vi "Autonomous Independent.vi"() -> ()   [LabVIEW 2020]
doc: "This VI is called when autonomous begins, and will automatically be terminated when autonomous ends. You can carry out timed or sensor driven robot movement independently without needing to return to the caller."
uses:
  <vilib>/Rock Robotics/WPI/ThirdParty/Phoenix-LabVIEW/Motor Controller/Controls/CTRE_Phoenix_MotorControl_ControlMode.ctl
  <vilib>/Rock Robotics/WPI/SafetyOutput/WPI_SafetyOutputConfigMenu.ctl
  <vilib>/Rock Robotics/WPI/Solenoid/WPI_SolenoidValue.ctl
  <vilib>/Rock Robotics/WPI/Utilities/WPI_GetSetVariantRefNum.vi
  <vilib>/Rock Robotics/Network Tables/NT Read String.vi
  <vilib>/Rock Robotics/Network Tables/NT Write Numeric Array.vi
  <vilib>/Rock Robotics/WPI/RobotDrive/WPI_RobotDriveMecanumDrive_Cartesian.vi
  <vilib>/Rock Robotics/WPI/Solenoid/WPI_SolenoidSetEnum.vi
panel:
  out "Current Movement, for debugging":T1={"X Joystick Value"=0.0, "Y Joystick Value"=-0.25, "Delay (sec)"=2.0, "Movement Name"="Drive Forwad", "Z Joystick Value "=0.0} {"Y Joystick Value" scale=1.0..-1.0; "X Joystick Value" scale=-1.0..1.0}
  in  "Array of robot movements":T2(array[cluster])=[{"X Joystick Value"=0.0, "Y Joystick Value"=0.25, "Delay (sec)"=1.0, "Movement Name"="Go Back", "Z Joystick Value"=0.0}, {"X Joystick Value"=0.0, "Y Joystick Value"=0.0, "Delay (sec)"=3.0, "Movement Name"="STOP", "Z Joystick Value"=0.0}, {"X Joystick Value"=0.0, "Y Joystick Value"=-0.25, "Delay (sec)"=2.0, "Movement Name"="Drive Forwad", "Z Joystick Value"=0.0}]
  # "Be sure to right-click and choose Data Operations>>Make Current Value default if you want to save the array values with the VI"
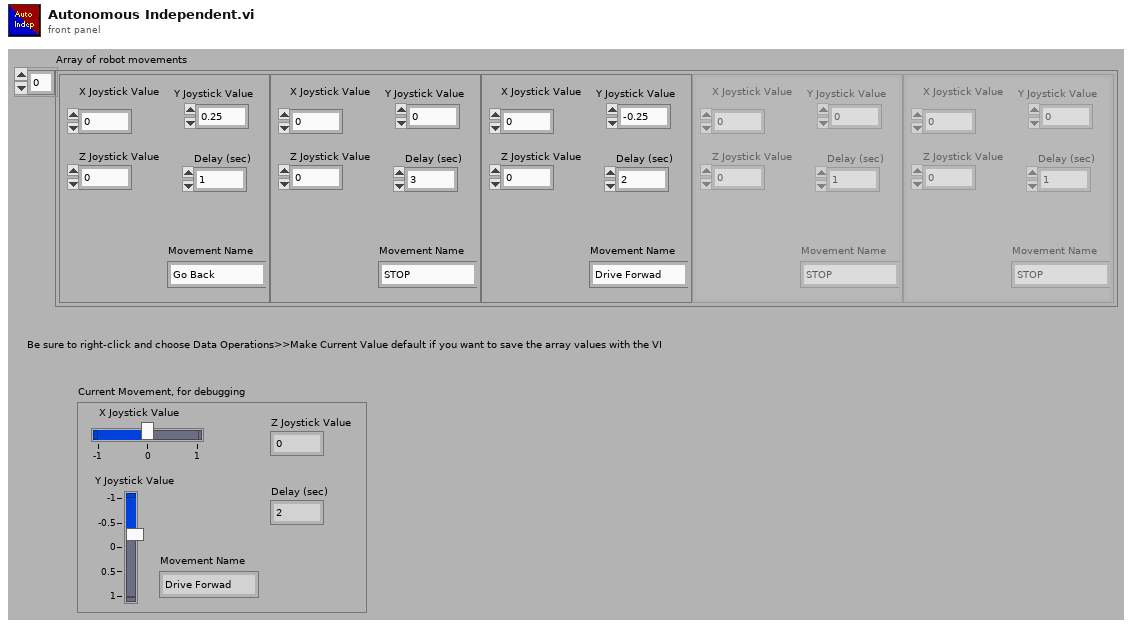
[diagram p1: front panel]
types:
  T1 = cluster{"X Joystick Value":dbl, "Y Joystick Value":dbl, "Delay (sec)":dbl, "Movement Name":string, "Z Joystick Value ":dbl}
  T2 = cluster{"X Joystick Value":dbl, "Y Joystick Value":dbl, "Delay (sec)":dbl, "Movement Name":string, "Z Joystick Value":dbl}[]
  T3 = typedef "WPI_JoystickDevRef.ctl" = cluster{"Device":T4}
  T4 = typedef "WPI_JoystickDeviceEnum.ctl" = enum16{"USB 0", "USB 1", "USB 2", "USB 3", "USB 4", "USB 5"}
  T5 = typedef "WPI_SafetyOutputConfigMenu.ctl" = enum16{"Enable", "Disable"}
  T6 = typedef "WPI_SolenoidValue.ctl" = enum16{"Off", "On", "Forward", "Reverse"}
  T7 = typedef "WPI_MotorControlDeviceRef.ctl" = cluster{"DeviceStatus":errorcluster, "Type":T8, "PWM":cluster{"PWM Channel":T9, "DeadBand":T10}, "CAN":cluster{"Device Number":u8, "SetOutput VI Ref":variant, "GetOutput VI Ref":variant, "Enable VI Ref":variant, "Disable VI Ref":variant, "Data":variant}, "Invert":bool, "DIO PWM":cluster{"PWM \"Enable\" Channel":T9, "DIOChannel":T11, "PWM Rate":dbl}}
  T8 = typedef "WPI_MotorControlType.ctl" = enum16{"PWM", "CAN", "DIO PWM"}
  T9 = typedef "FPGA_DIOPWMChannel.ctl" = enum8{"PWM 0", "PWM 1", "PWM 2", "PWM 3", "PWM 4", "PWM 5", "PWM 6", "PWM 7", "PWM 8", "PWM 9", "PWM MXP 0", "PWM MXP 1", "PWM MXP 2", "PWM MXP 3", "PWM MXP 4", "PWM MXP 5", "PWM MXP 6", "PWM MXP 7", "PWM MXP 8", "PWM MXP 9", "Invalid"}
  T10 = typedef "WPI_PWMDeadband.ctl" = cluster{"Name":string, "maxPositivePwm":i32, "minPositivePwm":i32, "centerPwm":i32, "maxNegativePwm":i32, "minNegativePwm":i32, "angularRange":u16}
  T11 = typedef "FPGA_DIOChannel.ctl" = enum8{"DIO 0", "DIO 1", "DIO 2", "DIO 3", "DIO 4", "DIO 5", "DIO 6", "DIO 7", "DIO 8", "DIO 9", "DIO MXP 0", "DIO MXP 1", "DIO MXP 2", "DIO MXP 3", "DIO MXP 4", "DIO MXP 5", "DIO MXP 6", "DIO MXP 7", "DIO MXP 8", "DIO MXP 9", "DIO MXP 10", "DIO MXP 11", "DIO MXP 12", "DIO MXP 13", "DIO MXP 14", "DIO MXP 15", "SPI Port CS1", "SPI Port CS2", "SPI Port CS3", "SPI Port MISO", "SPI Port MOSI", "Invalid"}
  T12 = typedef "WPI_RobotDriveDevRef.ctl" = cluster{"DevStatus":errorcluster, "Motors[]":T7[], "Square Inputs":bool, "Max Output":dbl}
  T13 = typedef "CTRE_Phoenix_MotorControl_ControlMode.ctl" = u16
  T14 = typedef "WPI_EncoderDevRef.ctl" = cluster{"DevStatus":errorcluster, "EncoderIndex":T15, "CounterIndex":T16, "DistancePerCount":dbl, "Decoding Type":T17}
  T15 = typedef "FPGA_EncoderIdx.ctl" = enum8{"Enc 0", "Enc 1", "Enc 2", "Enc 3", "Enc 4", "Enc 5", "Enc 6", "Enc 7", "Invalid"}
  T16 = typedef "FPGA_CounterCtrSystemIndex.ctl" = enum8{"Ctr 0", "Ctr 1", "Ctr 2", "Ctr 3", "Ctr 4", "Ctr 5", "Ctr 6", "Ctr 7", "Invalid"}
  T17 = typedef "WPI_EncoderType.ctl" = enum16{"1x", "2x", "4x"}
  T18 = typedef "WPI_SolenoidDevRef.ctl" = cluster{"DevStatus":errorcluster, "Pneumatics Control Module":u8, "Forward Solenoid Channel":T19, "Reverse Solenoid Channel":T19}
  T19 = typedef "WPI_SolenoidChannel.ctl" = enum8{"Solenoid 0", "Solenoid 1", "Solenoid 2", "Solenoid 3", "Solenoid 4", "Solenoid 5", "Solenoid 6", "Solenoid 7", "Solenoid 8", "Solenoid 9", "Solenoid 10", "Solenoid 11", "Solenoid 12", "Solenoid 13", "Solenoid 14", "Solenoid 15", "Invalid"}
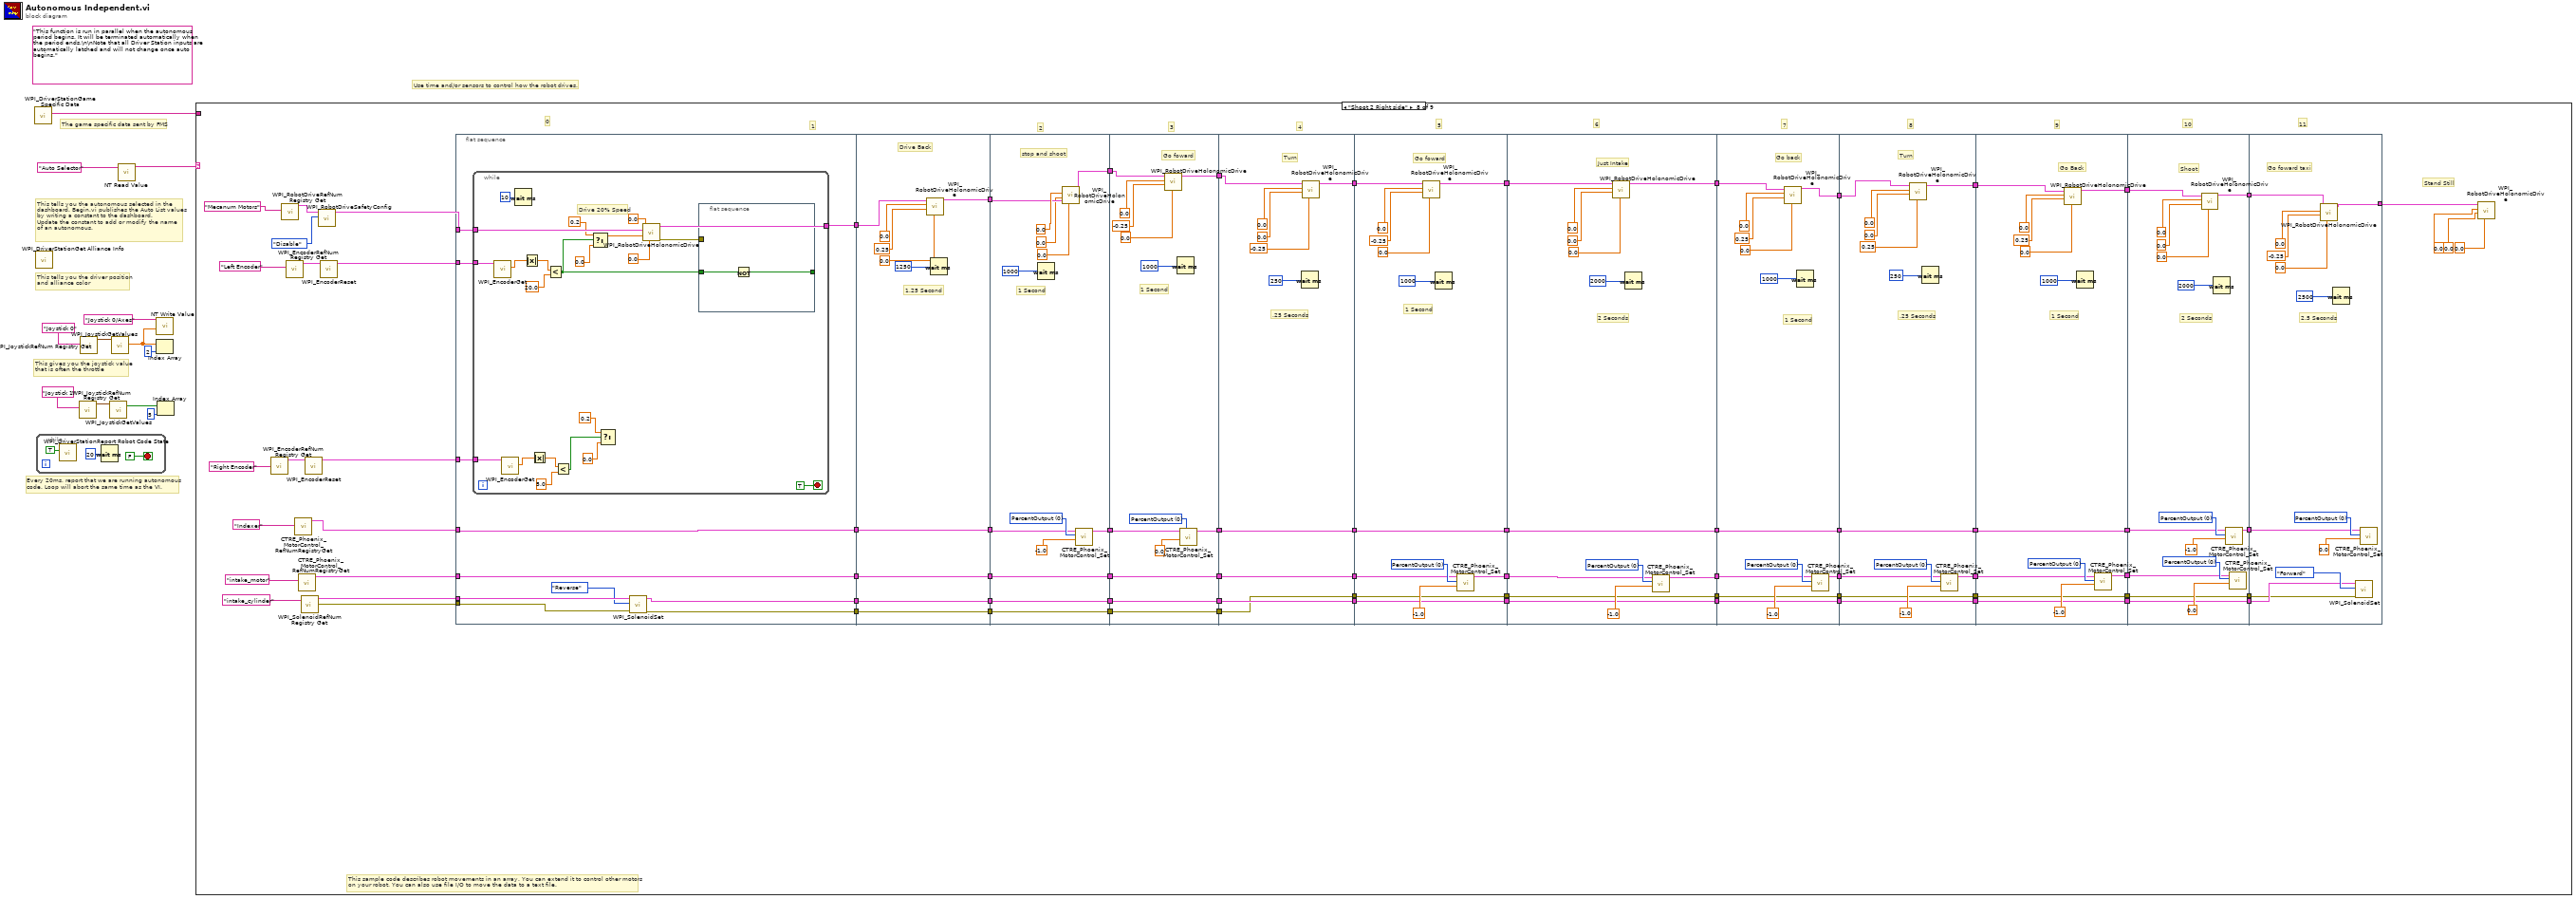
[diagram p0: block diagram]
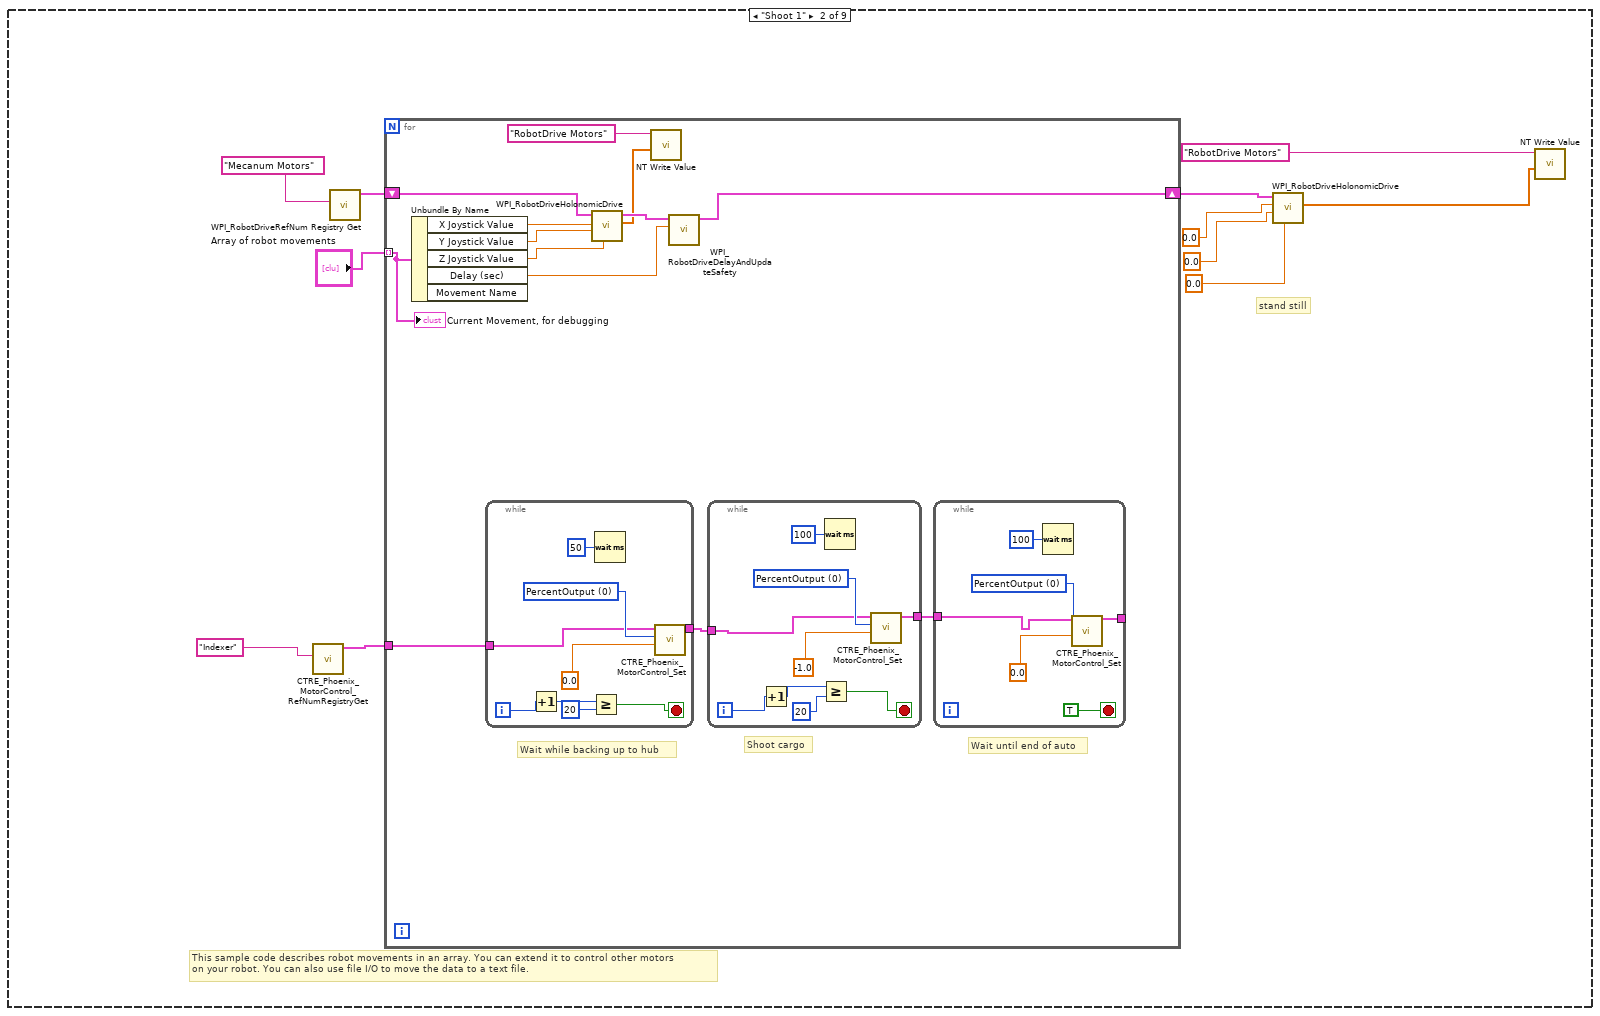
[diagram p3: hidden frame]
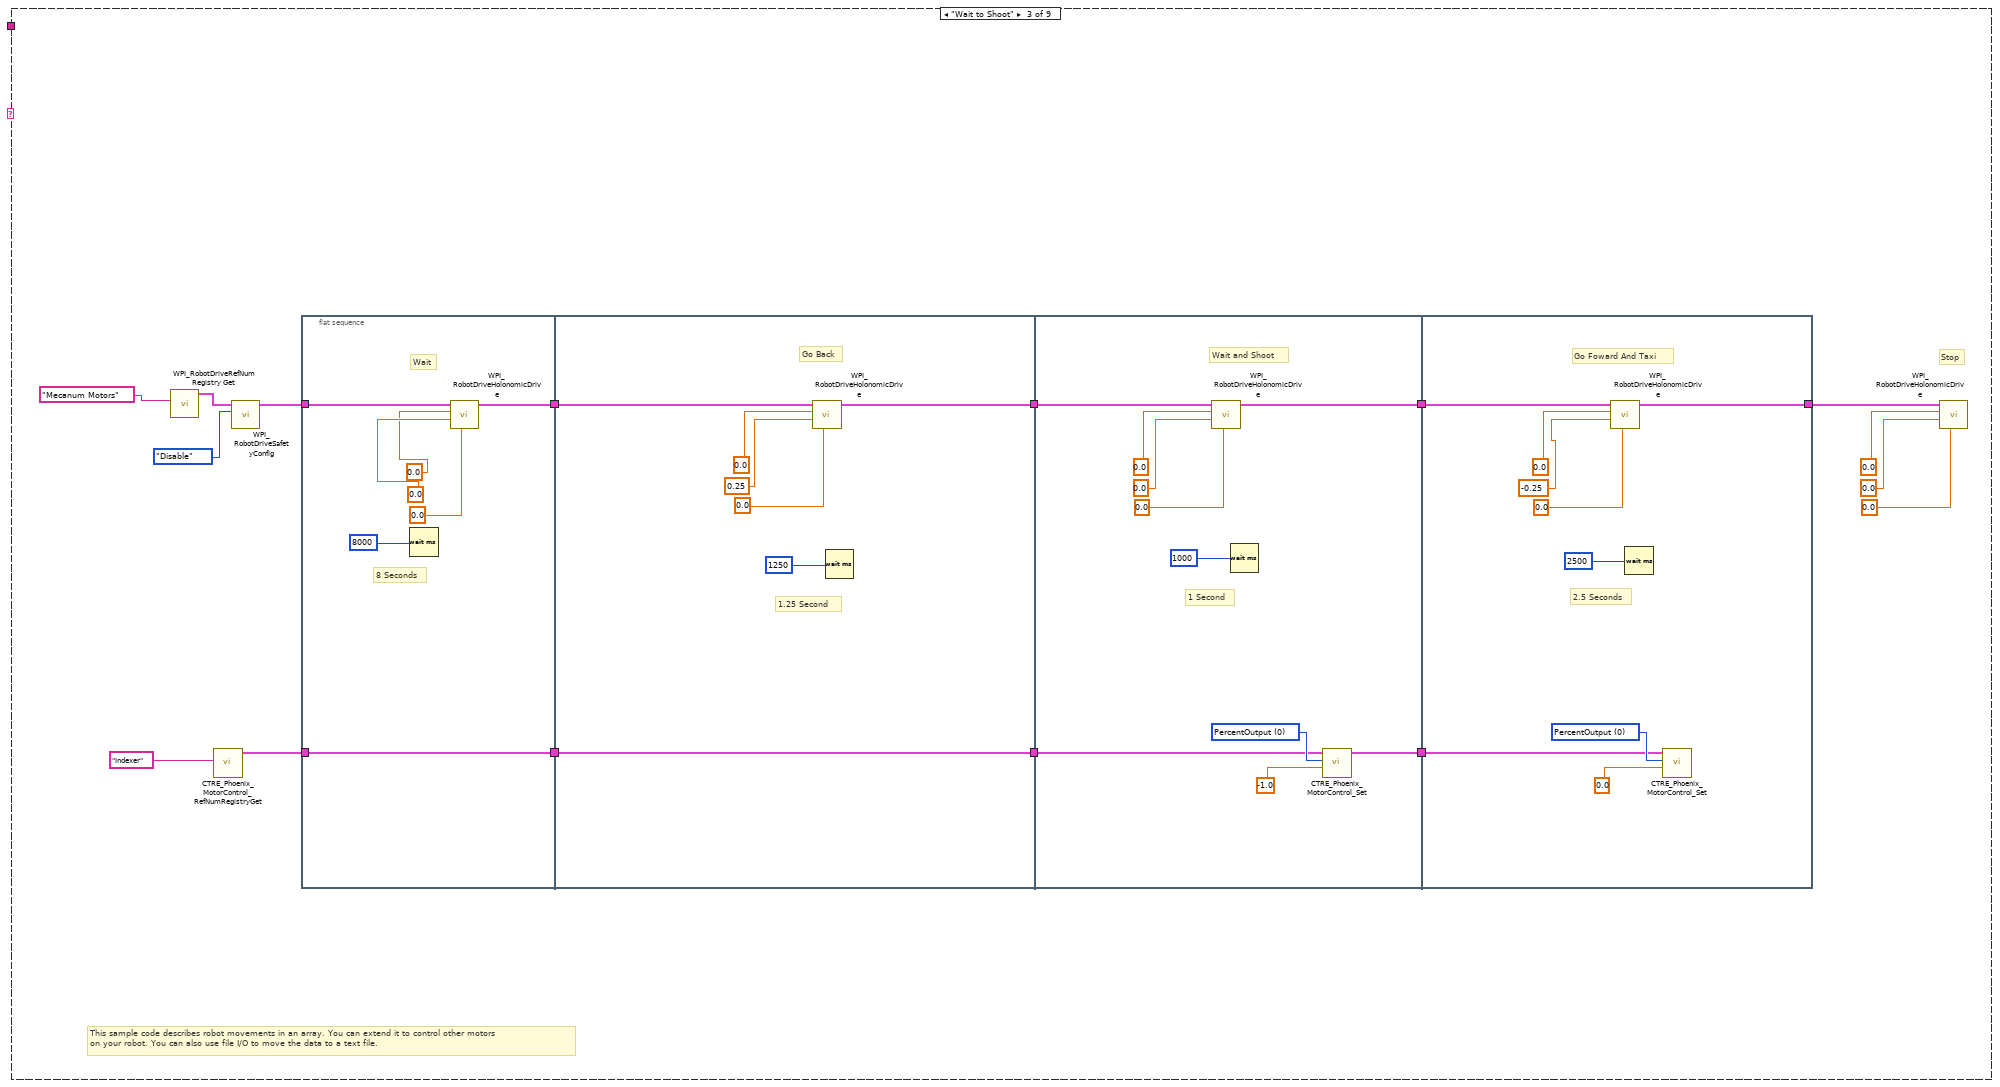
[diagram p4: hidden frame]
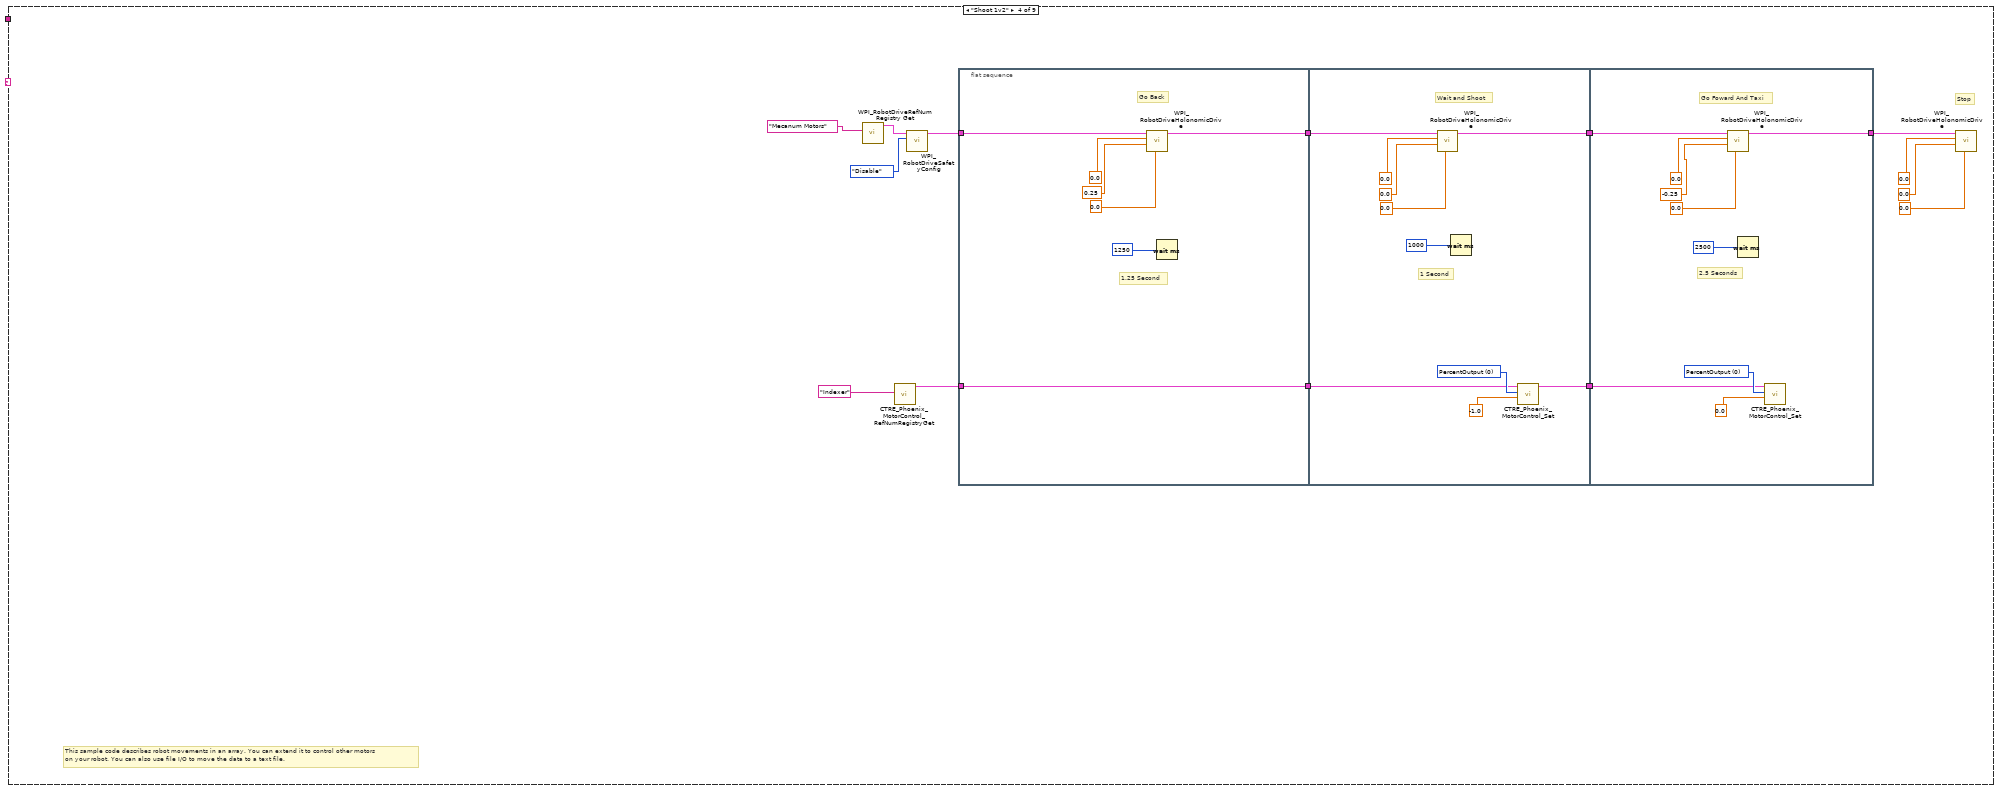
[diagram p5: hidden frame]
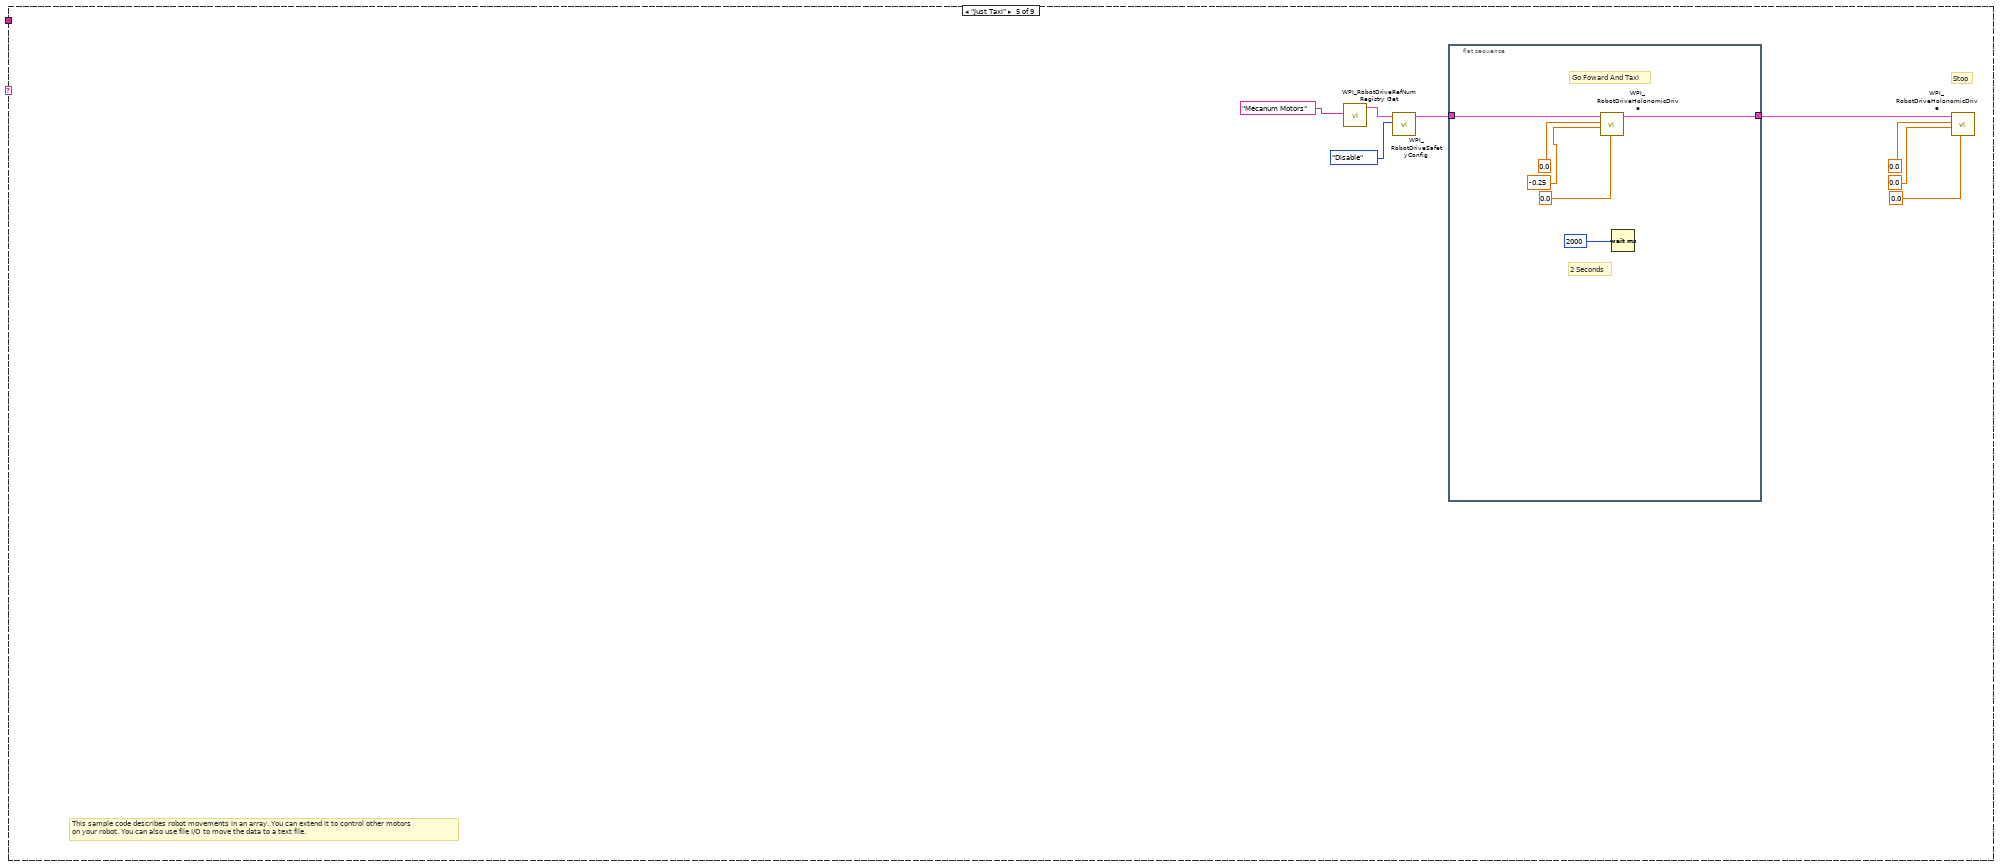
[diagram p6: hidden frame]
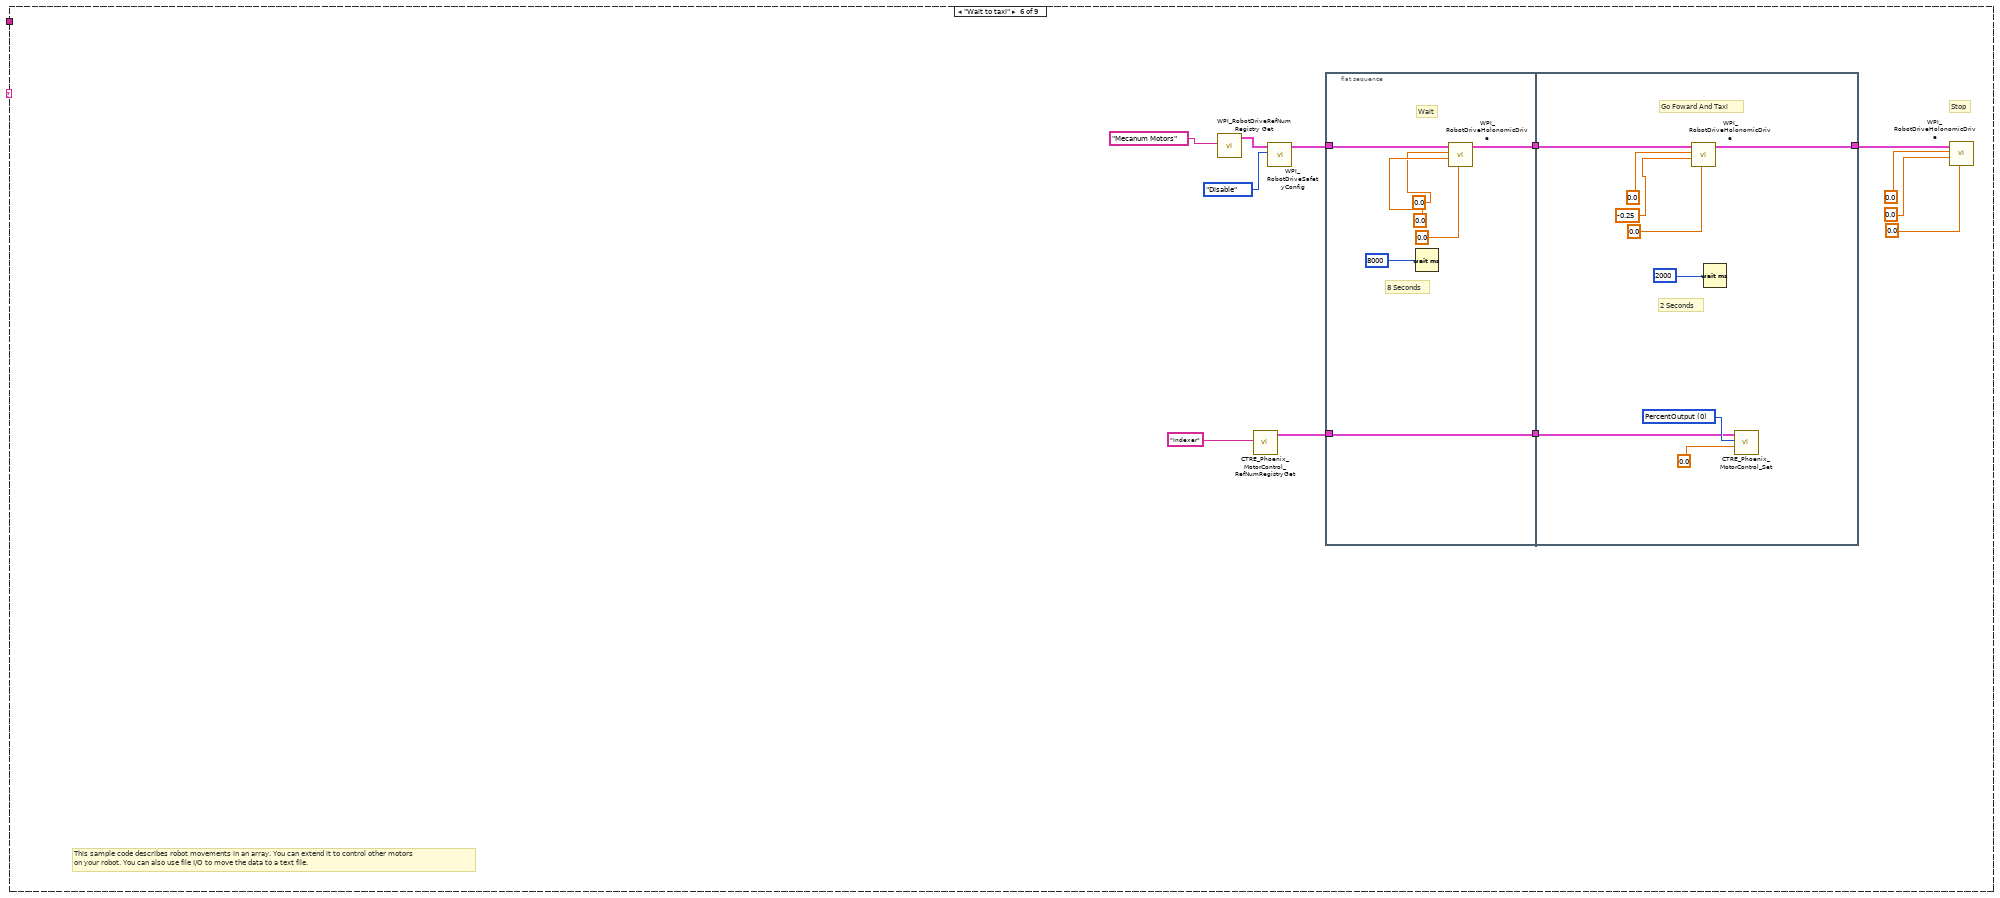
[diagram p7: hidden frame]
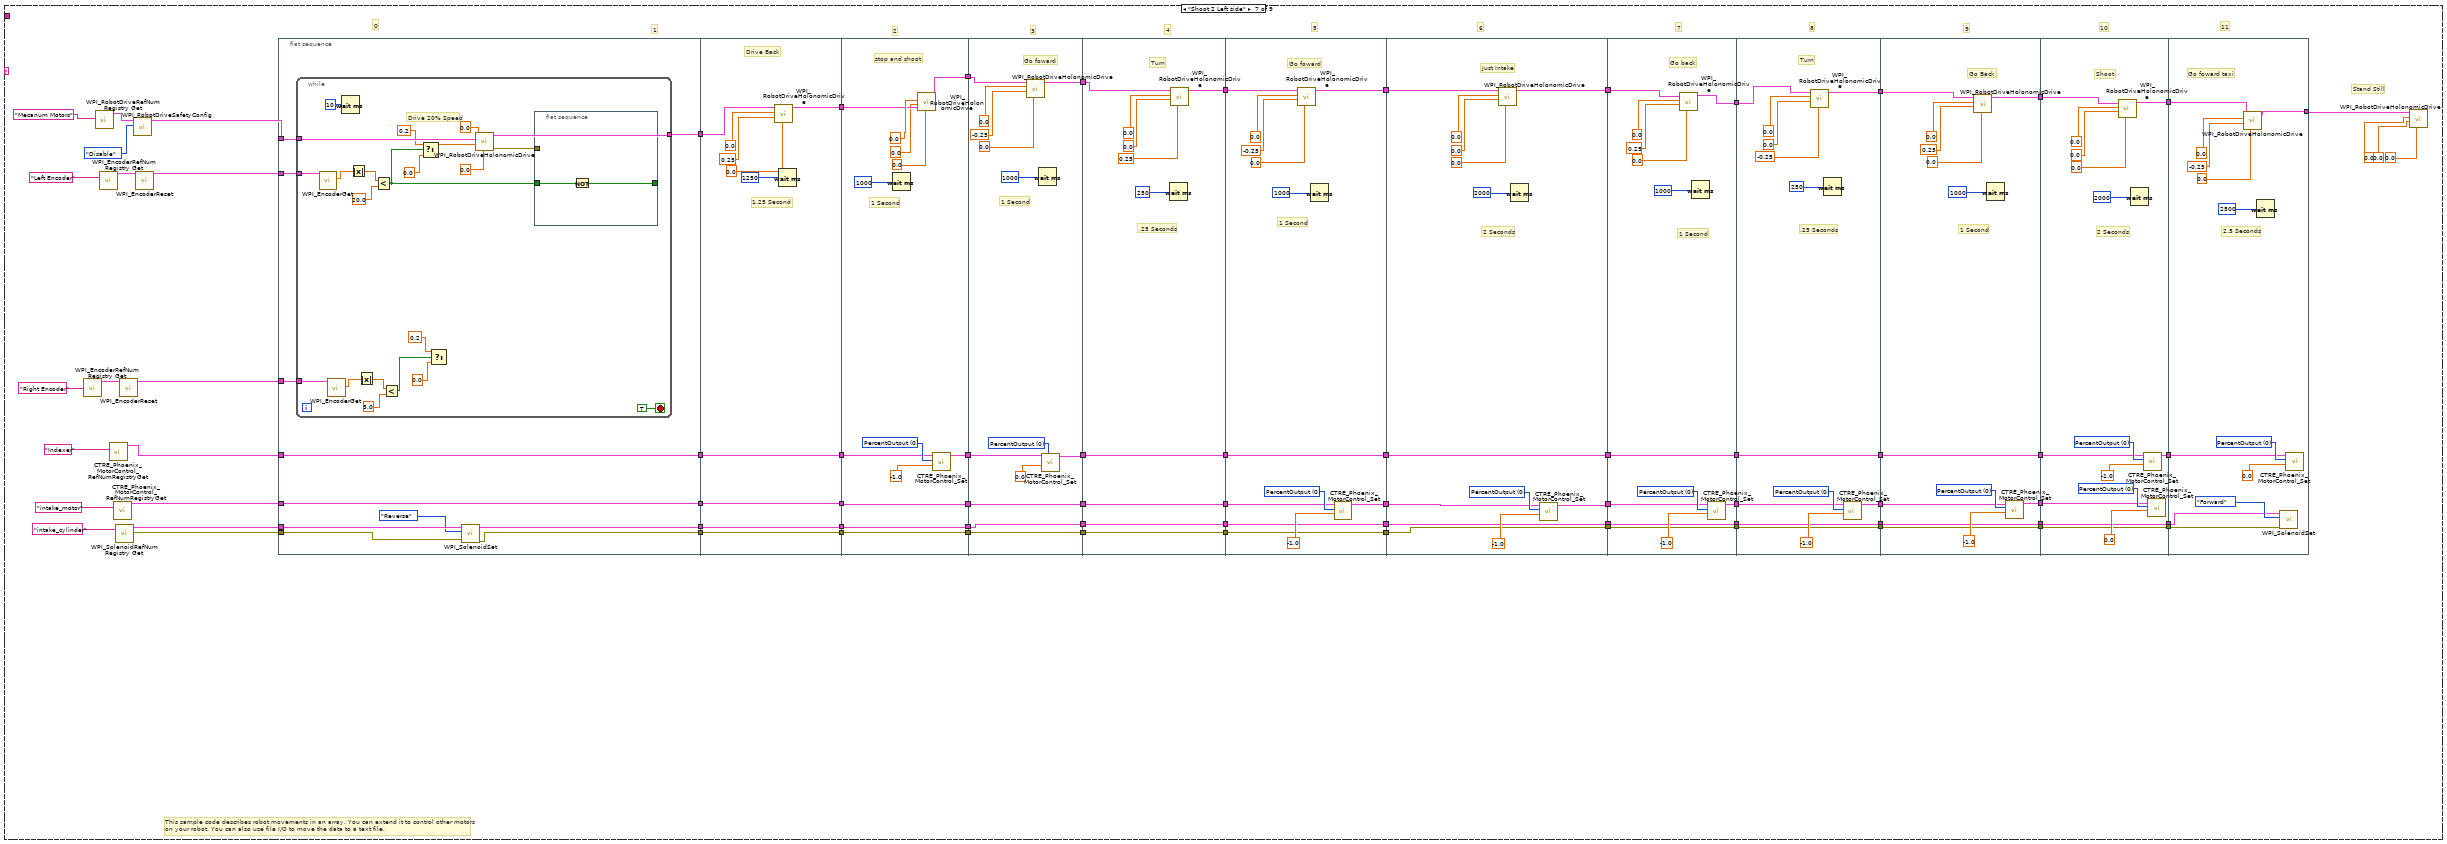
[diagram p8: hidden frame]
diagram:
  (unwired) "This function is run in parallel when the autonomous period begins. It will be terminated automatically when the period ends.\n\nNote that all Driver Station inputs are automatically latched and will not change once auto begins."
  # "The game specific data sent by FMS"
  # "This tells you the autonomous selected in the \ndashboard. Begin.vi publishes the Auto List values\nby writing a constant to the dashboard.\nUpdate the constant to add or modify the name\nof an autonomous."
  # "Every 20ms, report that we are running autonomous\ncode. Loop will abort the same time as the VI."
  # "This gives you the joystick value\nthat is often the throttle"
  # "Use time and/or sensors to control how the robot drives."
  # "This tells you the driver position\nand alliance color"
  n1 = call <vilib>:"WPI_DriverStationGame Specific Data.vi"() -> ("Game Specific Data"=w6:string)  [unwired: 11 in]
  n2 = call <vilib>:"WPI_DriverStationGet Alliance Info.vi"() -> ()  [unwired: 12 out]
  n3 = while {
    stop <- FALSE stop-if-true
    n4 = call <vilib>:"WPI_DriverStationReport Robot Code State.vi"("Autonomous"=TRUE) -> ()  [unwired: 10 in, 1 out]
    n5 = Wait (ms)(milliseconds to wait=u32 20) -> ()  [unwired: 1 out]
  }
  n6 = call <vilib>:"WPI_JoystickRefNum Registry Get.vi"("refnum name"="Joystick 1") -> ("JoystickDevRef"=w5:T3)  [unwired: 1 in, 9 out]
  n7 = call <vilib>:"WPI_JoystickRefNum Registry Get.vi"("refnum name"="Joystick 0") -> ("JoystickDevRef"=w11:T3)  [unwired: 1 in, 9 out]
  n8 = call <vilib>:"WPI_JoystickGetValues.vi"("JoystickDevRef"=w5) -> ("Buttons"=w1:bool[])  [unwired: 6 in, 4 out]
  n9 = call <vilib>:"WPI_JoystickGetValues.vi"("JoystickDevRef"=w11) -> ("Axes"=w8:dbl[])  [unwired: 6 in, 4 out]
  n10 = call-poly <vilib>:"NT Read Value.vi"("Name"="Auto Selector") -> ("String"=w2:string)  [unwired: 9 in, 1 out]
  n11 = call-poly <vilib>:"NT Write Value.vi"("Numeric Array"=w8, "Name"="Joystick 0/Axes") -> ()  [unwired: 9 in, 1 out]
  n12 = Index Array(array=w8, index=2) -> ()  [unwired: 1 out]
  n13 = Index Array(array=w1, index=5) -> ()  [unwired: 1 out]
  n14 = case shown="\"Shoot 2 Right side\"" w2 {
    tunnel: w6 -> [_ _ _ _ _ _ _ _ _]
    frame Default {
      # "You can put your main auto here, or you can right-click on the case and make any\nother frame be the default case."
      # "This is the frame that will execute if no selection is made, or if it is not recognized"
    }
    frame "Shoot 1" {
      # "stand still"
      # "This sample code describes robot movements in an array. You can extend it to control other motors\non your robot. You can also use file I/O to move the data to a text file."
      n15 = call <vilib>:"CTRE_Phoenix_MotorControl_RefNumRegistryGet.vi"("refnum name"="Indexer") -> ("PhoenixMotorControlDevRef"=w16:T7)  [unwired: 9 in, 1 out]
      n16 = call <vilib>:"WPI_RobotDriveRefNum Registry Get.vi"("refnum name"="Mecanum Motors") -> ("RobotDriveDevRef"=w26:T12)  [unwired: 1 in, 9 out]
      n17 = for {
        shift-right: [w38] -> w22
        shift-left: w26 -> [w30]
        tunnel: "Array of robot movements" -> [w34] mode=indexing
        tunnel: w16 -> [w29]
        # "Wait until end of auto"
        # "Shoot cargo"
        # "Wait while backing up to hub"
        n18 = Unbundle By Name "Unbundle By Name"(w34) -> ("X Joystick Value"=w37:dbl, "Y Joystick Value"=w36:dbl, "Z Joystick Value"=w31:dbl, "Delay (sec)"=w35:dbl)  [unwired: 1 out]
        n19 = while {
          tunnel: w29 -> [w62]
          tunnel: [w55] -> w28
          i -> [w60]
          stop <- w58 stop-if-true
          w63 = T13 0 items=["PercentOutput"=0, "Position"=1, "Velocity"=2, "Current"=3, "Follower"=5, "MotionProfile"=6, "MotionMagic"=7, "MotionProfileArc"=10, "Disabled"=15] ("Control Mode")
          n20 = Increment(x=w60) -> (x+1=w59:i32)
          n21 = Greater Or Equal?(x=w59, y=20) -> (x >= y?=w58:bool)
          n22 = Wait (ms)(milliseconds to wait=u32 50) -> ()  [unwired: 1 out]
          n23 = call <vilib>:"CTRE_Phoenix_MotorControl_Set.vi"("Output"=0.0, "Control Mode"=w63, "PhoenixMotorControlDevRef"=w62) -> ("PhoenixMotorControlDevRef"=w55:T7)  [unwired: 7 in, 1 out]
        }
        n24 = call-poly <vilib>:"WPI_RobotDriveHolonomicDrive.vi"("Rotation"=w31, "Y"=w36, "X"=w37, "RobotDriveDevRef"=w30) -> ("Motor Values"=w32:dbl[], "RobotDriveDevRef"=w39:T12)  [unwired: 5 in, 1 out]
        n25 = call-poly <vilib>:"NT Write Value.vi"("Numeric Array"=w32, "Name"="RobotDrive Motors") -> ()  [unwired: 9 in, 1 out]
        n26 = call <vilib>:"WPI_RobotDriveDelayAndUpdateSafety.vi"("Delay (s)"=w35, "RobotDriveDevRef"=w39) -> ("RobotDriveDevRef 2"=w38:T12)  [unwired: 8 in, 1 out]
        n27 = while {
          tunnel: w28 -> [w50]
          tunnel: [w47] -> w27
          i -> [w49]
          stop <- w48 stop-if-true
          w54 = T13 0 items=["PercentOutput"=0, "Position"=1, "Velocity"=2, "Current"=3, "Follower"=5, "MotionProfile"=6, "MotionMagic"=7, "MotionProfileArc"=10, "Disabled"=15] ("Control Mode")
          n28 = Increment(x=w49) -> (x+1=w46:i32)
          n29 = Greater Or Equal?(x=w46, y=20) -> (x >= y?=w48:bool)
          n30 = Wait (ms)(milliseconds to wait=u32 100) -> ()  [unwired: 1 out]
          n31 = call <vilib>:"CTRE_Phoenix_MotorControl_Set.vi"("Output"=-1.0, "Control Mode"=w54, "PhoenixMotorControlDevRef"=w50) -> ("PhoenixMotorControlDevRef"=w47:T7)  [unwired: 7 in, 1 out]
        }
        n32 = while {
          tunnel: w27 -> [w42]
          tunnel: [w41] -> _
          stop <- TRUE stop-if-true
          w45 = T13 0 items=["PercentOutput"=0, "Position"=1, "Velocity"=2, "Current"=3, "Follower"=5, "MotionProfile"=6, "MotionMagic"=7, "MotionProfileArc"=10, "Disabled"=15] ("Control Mode")
          n33 = Wait (ms)(milliseconds to wait=u32 100) -> ()  [unwired: 1 out]
          n34 = call <vilib>:"CTRE_Phoenix_MotorControl_Set.vi"("Output"=0.0, "Control Mode"=w45, "PhoenixMotorControlDevRef"=w42) -> ("PhoenixMotorControlDevRef"=w41:T7)  [unwired: 7 in, 1 out]
        }
        "Current Movement, for debugging" <- w34
      }
      n35 = call-poly <vilib>:"WPI_RobotDriveHolonomicDrive.vi"("Rotation"=0.0 ("X axis value"), "Y"=0.0 ("X axis value"), "X"=0.0 ("X axis value"), "RobotDriveDevRef"=w22) -> ("Motor Values"=w19:dbl[])  [unwired: 5 in, 2 out]
      n36 = call-poly <vilib>:"NT Write Value.vi"("Numeric Array"=w19, "Name"="RobotDrive Motors") -> ()  [unwired: 9 in, 1 out]
    }
    frame "Wait to Shoot" {
      # "Stop"
      # "This sample code describes robot movements in an array. You can extend it to control other motors\non your robot. You can also use file I/O to move the data to a text file."
      n37 = call <vilib>:"WPI_RobotDriveRefNum Registry Get.vi"("refnum name"="Mecanum Motors") -> ("RobotDriveDevRef"=w77:T12)  [unwired: 1 in, 9 out]
      n38 = call <vilib>:"CTRE_Phoenix_MotorControl_RefNumRegistryGet.vi"("refnum name"="Indexer") -> ("PhoenixMotorControlDevRef"=w64:T7)  [unwired: 9 in, 1 out]
      n39 = call <vilib>:"WPI_RobotDriveSafetyConfig.vi"("mode"=WPI_SafetyOutputConfigMenu."Disable", "RobotDriveDevRef"=w77) -> ("RobotDriveDevRef"=w76:T12)  [unwired: 8 in, 1 out]
      n40 = flat-sequence {
        tunnel: w76 -> [w82]
        tunnel: [w81] -> w75
        tunnel: [w80] -> w65
        tunnel: w64 -> [w80]
        tunnel: w75 -> [w89]
        tunnel: [w88] -> w74
        tunnel: [w87] -> w66
        tunnel: w65 -> [w87]
        tunnel: w74 -> [w99]
        tunnel: [w98] -> w73
        tunnel: [w95] -> w67
        tunnel: w66 -> [w94]
        tunnel: w73 -> [w110]
        tunnel: [w109] -> w69
        tunnel: w67 -> [w106]
        frame #0 {
          # "Wait"
          # "8 Seconds"
          n41 = Wait (ms)(milliseconds to wait=u32 8000) -> ()  [unwired: 1 out]
          n42 = call-poly <vilib>:"WPI_RobotDriveHolonomicDrive.vi"("Rotation"=0.0 ("X axis value"), "Y"=0.0 ("X axis value"), "X"=0.0 ("X axis value"), "RobotDriveDevRef"=w82) -> ("RobotDriveDevRef"=w81:T12)  [unwired: 5 in, 2 out]
        }
        frame #1 {
          # "Go Back"
          # "1.25 Second"
          n43 = call-poly <vilib>:"WPI_RobotDriveHolonomicDrive.vi"("Rotation"=0.0, "Y"=0.25, "X"=0.0, "RobotDriveDevRef"=w89) -> ("RobotDriveDevRef"=w88:T12)  [unwired: 5 in, 2 out]
          n44 = Wait (ms)(milliseconds to wait=u32 1250) -> ()  [unwired: 1 out]
        }
        frame #2 {
          w97 = T13 0 items=["PercentOutput"=0, "Position"=1, "Velocity"=2, "Current"=3, "Follower"=5, "MotionProfile"=6, "MotionMagic"=7, "MotionProfileArc"=10, "Disabled"=15] ("Control Mode")
          # "Wait and Shoot"
          # "1 Second"
          n45 = call-poly <vilib>:"WPI_RobotDriveHolonomicDrive.vi"("Rotation"=0.0, "Y"=0.0, "X"=0.0, "RobotDriveDevRef"=w99) -> ("RobotDriveDevRef"=w98:T12)  [unwired: 5 in, 2 out]
          n46 = Wait (ms)(milliseconds to wait=u32 1000) -> ()  [unwired: 1 out]
          n47 = call <vilib>:"CTRE_Phoenix_MotorControl_Set.vi"("Output"=-1.0, "Control Mode"=w97, "PhoenixMotorControlDevRef"=w94) -> ("PhoenixMotorControlDevRef"=w95:T7)  [unwired: 7 in, 1 out]
        }
        frame #3 {
          w108 = T13 0 items=["PercentOutput"=0, "Position"=1, "Velocity"=2, "Current"=3, "Follower"=5, "MotionProfile"=6, "MotionMagic"=7, "MotionProfileArc"=10, "Disabled"=15] ("Control Mode")
          # "2.5 Seconds"
          # "Go Foward And Taxi"
          n48 = call-poly <vilib>:"WPI_RobotDriveHolonomicDrive.vi"("Rotation"=0.0, "Y"=-0.25, "X"=0.0, "RobotDriveDevRef"=w110) -> ("RobotDriveDevRef"=w109:T12)  [unwired: 5 in, 2 out]
          n49 = Wait (ms)(milliseconds to wait=u32 2500) -> ()  [unwired: 1 out]
          n50 = call <vilib>:"CTRE_Phoenix_MotorControl_Set.vi"("Output"=0.0, "Control Mode"=w108, "PhoenixMotorControlDevRef"=w106) -> ()  [unwired: 7 in, 2 out]
        }
      }
      n51 = call-poly <vilib>:"WPI_RobotDriveHolonomicDrive.vi"("Rotation"=0.0, "Y"=0.0, "X"=0.0, "RobotDriveDevRef"=w69) -> ()  [unwired: 5 in, 3 out]
    }
    frame "Shoot 1v2" {
      # "Stop"
      # "This sample code describes robot movements in an array. You can extend it to control other motors\non your robot. You can also use file I/O to move the data to a text file."
      n52 = call <vilib>:"WPI_RobotDriveRefNum Registry Get.vi"("refnum name"="Mecanum Motors") -> ("RobotDriveDevRef"=w124:T12)  [unwired: 1 in, 9 out]
      n53 = call <vilib>:"CTRE_Phoenix_MotorControl_RefNumRegistryGet.vi"("refnum name"="Indexer") -> ("PhoenixMotorControlDevRef"=w114:T7)  [unwired: 9 in, 1 out]
      n54 = call <vilib>:"WPI_RobotDriveSafetyConfig.vi"("mode"=WPI_SafetyOutputConfigMenu."Disable", "RobotDriveDevRef"=w124) -> ("RobotDriveDevRef"=w113:T12)  [unwired: 8 in, 1 out]
      n55 = flat-sequence {
        tunnel: [w129] -> w123
        tunnel: [w128] -> w115
        tunnel: w114 -> [w128]
        tunnel: w113 -> [w127]
        tunnel: w123 -> [w139]
        tunnel: [w138] -> w122
        tunnel: [w135] -> w116
        tunnel: w115 -> [w134]
        tunnel: w122 -> [w150]
        tunnel: [w149] -> w118
        tunnel: w116 -> [w146]
        frame #0 {
          # "Go Back"
          # "1.25 Second"
          n56 = call-poly <vilib>:"WPI_RobotDriveHolonomicDrive.vi"("Rotation"=0.0, "Y"=0.25, "X"=0.0, "RobotDriveDevRef"=w127) -> ("RobotDriveDevRef"=w129:T12)  [unwired: 5 in, 2 out]
          n57 = Wait (ms)(milliseconds to wait=u32 1250) -> ()  [unwired: 1 out]
        }
        frame #1 {
          w137 = T13 0 items=["PercentOutput"=0, "Position"=1, "Velocity"=2, "Current"=3, "Follower"=5, "MotionProfile"=6, "MotionMagic"=7, "MotionProfileArc"=10, "Disabled"=15] ("Control Mode")
          # "Wait and Shoot"
          # "1 Second"
          n58 = call-poly <vilib>:"WPI_RobotDriveHolonomicDrive.vi"("Rotation"=0.0, "Y"=0.0, "X"=0.0, "RobotDriveDevRef"=w139) -> ("RobotDriveDevRef"=w138:T12)  [unwired: 5 in, 2 out]
          n59 = Wait (ms)(milliseconds to wait=u32 1000) -> ()  [unwired: 1 out]
          n60 = call <vilib>:"CTRE_Phoenix_MotorControl_Set.vi"("Output"=-1.0, "Control Mode"=w137, "PhoenixMotorControlDevRef"=w134) -> ("PhoenixMotorControlDevRef"=w135:T7)  [unwired: 7 in, 1 out]
        }
        frame #2 {
          w148 = T13 0 items=["PercentOutput"=0, "Position"=1, "Velocity"=2, "Current"=3, "Follower"=5, "MotionProfile"=6, "MotionMagic"=7, "MotionProfileArc"=10, "Disabled"=15] ("Control Mode")
          # "2.5 Seconds"
          # "Go Foward And Taxi"
          n61 = call-poly <vilib>:"WPI_RobotDriveHolonomicDrive.vi"("Rotation"=0.0, "Y"=-0.25, "X"=0.0, "RobotDriveDevRef"=w150) -> ("RobotDriveDevRef"=w149:T12)  [unwired: 5 in, 2 out]
          n62 = Wait (ms)(milliseconds to wait=u32 2500) -> ()  [unwired: 1 out]
          n63 = call <vilib>:"CTRE_Phoenix_MotorControl_Set.vi"("Output"=0.0, "Control Mode"=w148, "PhoenixMotorControlDevRef"=w146) -> ()  [unwired: 7 in, 2 out]
        }
      }
      n64 = call-poly <vilib>:"WPI_RobotDriveHolonomicDrive.vi"("Rotation"=0.0, "Y"=0.0, "X"=0.0, "RobotDriveDevRef"=w118) -> ()  [unwired: 5 in, 3 out]
    }
    frame "Just Taxi" {
      # "Stop"
      # "This sample code describes robot movements in an array. You can extend it to control other motors\non your robot. You can also use file I/O to move the data to a text file."
      n65 = call <vilib>:"WPI_RobotDriveRefNum Registry Get.vi"("refnum name"="Mecanum Motors") -> ("RobotDriveDevRef"=w158:T12)  [unwired: 1 in, 9 out]
      n66 = call <vilib>:"WPI_RobotDriveSafetyConfig.vi"("mode"=WPI_SafetyOutputConfigMenu."Disable", "RobotDriveDevRef"=w158) -> ("RobotDriveDevRef"=w153:T12)  [unwired: 8 in, 1 out]
      n67 = flat-sequence {
        tunnel: [w164] -> w154
        tunnel: w153 -> [w161]
        frame #0 {
          # "2 Seconds"
          # "Go Foward And Taxi"
          n68 = call-poly <vilib>:"WPI_RobotDriveHolonomicDrive.vi"("Rotation"=0.0, "Y"=-0.25, "X"=0.0, "RobotDriveDevRef"=w161) -> ("RobotDriveDevRef"=w164:T12)  [unwired: 5 in, 2 out]
          n69 = Wait (ms)(milliseconds to wait=u32 2000) -> ()  [unwired: 1 out]
        }
      }
      n70 = call-poly <vilib>:"WPI_RobotDriveHolonomicDrive.vi"("Rotation"=0.0, "Y"=0.0, "X"=0.0, "RobotDriveDevRef"=w154) -> ()  [unwired: 5 in, 3 out]
    }
    frame "Wait to taxi" {
      # "Stop"
      # "This sample code describes robot movements in an array. You can extend it to control other motors\non your robot. You can also use file I/O to move the data to a text file."
      n71 = call <vilib>:"WPI_RobotDriveRefNum Registry Get.vi"("refnum name"="Mecanum Motors") -> ("RobotDriveDevRef"=w176:T12)  [unwired: 1 in, 9 out]
      n72 = call <vilib>:"CTRE_Phoenix_MotorControl_RefNumRegistryGet.vi"("refnum name"="Indexer") -> ("PhoenixMotorControlDevRef"=w169:T7)  [unwired: 9 in, 1 out]
      n73 = call <vilib>:"WPI_RobotDriveSafetyConfig.vi"("mode"=WPI_SafetyOutputConfigMenu."Disable", "RobotDriveDevRef"=w176) -> ("RobotDriveDevRef"=w175:T12)  [unwired: 8 in, 1 out]
      n74 = flat-sequence {
        tunnel: w175 -> [w181]
        tunnel: w169 -> [w179]
        tunnel: [w180] -> w168
        tunnel: [w179] -> w167
        tunnel: [w192] -> w171
        tunnel: w168 -> [w187]
        tunnel: w167 -> [w186]
        frame #0 {
          # "Wait"
          # "8 Seconds"
          n75 = Wait (ms)(milliseconds to wait=u32 8000) -> ()  [unwired: 1 out]
          n76 = call-poly <vilib>:"WPI_RobotDriveHolonomicDrive.vi"("Rotation"=0.0 ("X axis value"), "Y"=0.0 ("X axis value"), "X"=0.0 ("X axis value"), "RobotDriveDevRef"=w181) -> ("RobotDriveDevRef"=w180:T12)  [unwired: 5 in, 2 out]
        }
        frame #1 {
          w191 = T13 0 items=["PercentOutput"=0, "Position"=1, "Velocity"=2, "Current"=3, "Follower"=5, "MotionProfile"=6, "MotionMagic"=7, "MotionProfileArc"=10, "Disabled"=15] ("Control Mode")
          # "2 Seconds"
          # "Go Foward And Taxi"
          n77 = call-poly <vilib>:"WPI_RobotDriveHolonomicDrive.vi"("Rotation"=0.0, "Y"=-0.25, "X"=0.0, "RobotDriveDevRef"=w187) -> ("RobotDriveDevRef"=w192:T12)  [unwired: 5 in, 2 out]
          n78 = Wait (ms)(milliseconds to wait=u32 2000) -> ()  [unwired: 1 out]
          n79 = call <vilib>:"CTRE_Phoenix_MotorControl_Set.vi"("Output"=0.0, "Control Mode"=w191, "PhoenixMotorControlDevRef"=w186) -> ()  [unwired: 7 in, 2 out]
        }
      }
      n80 = call-poly <vilib>:"WPI_RobotDriveHolonomicDrive.vi"("Rotation"=0.0, "Y"=0.0, "X"=0.0, "RobotDriveDevRef"=w171) -> ()  [unwired: 5 in, 3 out]
    }
    frame "Shoot 2 Left side" {
      # "11"
      # "0"
      # "Stand Still"
      # "10"
      # "9"
      # "8"
      # "7"
      # "6"
      # "5"
      # "4"
      # "3"
      # "2"
      # "1"
      # "This sample code describes robot movements in an array. You can extend it to control other motors\non your robot. You can also use file I/O to move the data to a text file."
      n81 = call <vilib>:"WPI_EncoderRefNum Registry Get.vi"("refnum name"="Right Encoder") -> ("EncoderDevRef"=w235:T14)  [unwired: 9 in, 1 out]
      n82 = call <vilib>:"WPI_RobotDriveRefNum Registry Get.vi"("refnum name"="Mecanum Motors") -> ("RobotDriveDevRef"=w238:T12)  [unwired: 1 in, 9 out]
      n83 = call <vilib>:"WPI_EncoderRefNum Registry Get.vi"("refnum name"="Left Encoder") -> ("EncoderDevRef"=w243:T14)  [unwired: 9 in, 1 out]
      n84 = call <vilib>:"CTRE_Phoenix_MotorControl_RefNumRegistryGet.vi"("refnum name"="Indexer") -> ("PhoenixMotorControlDevRef"=w265:T7)  [unwired: 9 in, 1 out]
      n85 = call <vilib>:"CTRE_Phoenix_MotorControl_RefNumRegistryGet.vi"("refnum name"="intake_motor") -> ("PhoenixMotorControlDevRef"=w262:T7)  [unwired: 9 in, 1 out]
      n86 = call <vilib>:"WPI_SolenoidRefNum Registry Get.vi"("refnum name"="intake_cylinder") -> ("error out"=w227:errorcluster, "SolenoidDevRef"=w225:T18)  [unwired: 9 in]
      n87 = call <vilib>:"WPI_EncoderReset.vi"("EncoderDevRef"=w235) -> ("EncoderDevRef"=w234:T14)  [unwired: 9 in, 1 out]
      n88 = call <vilib>:"WPI_RobotDriveSafetyConfig.vi"("mode"=WPI_SafetyOutputConfigMenu."Disable", "RobotDriveDevRef"=w238) -> ("RobotDriveDevRef"=w237:T12)  [unwired: 8 in, 1 out]
      n89 = call <vilib>:"WPI_EncoderReset.vi"("EncoderDevRef"=w243) -> ("EncoderDevRef"=w242:T14)  [unwired: 9 in, 1 out]
      n90 = flat-sequence {
        tunnel: w262 -> [w279]
        tunnel: w265 -> [w280]
        tunnel: [w276] -> w246
        tunnel: [w280] -> w245
        tunnel: [w279] -> w244
        tunnel: w242 -> [w278]
        tunnel: w237 -> [w277]
        tunnel: w234 -> [w275]
        tunnel: w227 -> [w274]
        tunnel: w225 -> [w273]
        tunnel: [w271] -> w206
        tunnel: [w270] -> w205
        tunnel: [w310] -> w269
        tunnel: [w308] -> w266
        tunnel: [w307] -> w263
        tunnel: w246 -> [w313]
        tunnel: w245 -> [w308]
        tunnel: w244 -> [w307]
        tunnel: [w306] -> w207
        tunnel: w206 -> [w306]
        tunnel: w205 -> [w305]
        tunnel: [w305] -> w204
        tunnel: w269 -> [w324]
        tunnel: [w323] -> w268
        tunnel: w266 -> [w319]
        tunnel: w263 -> [w317]
        tunnel: [w318] -> w250
        tunnel: [w317] -> w247
        tunnel: [w316] -> w208
        tunnel: w207 -> [w316]
        tunnel: w204 -> [w315]
        tunnel: [w315] -> w203
        tunnel: w268 -> [w337]
        tunnel: [w335] -> w261
        tunnel: [w330] -> w251
        tunnel: w250 -> [w331]
        tunnel: [w334] -> w248
        tunnel: w247 -> [w334]
        tunnel: [w329] -> w209
        tunnel: w208 -> [w329]
        tunnel: w203 -> [w328]
        tunnel: [w328] -> w202
        tunnel: w261 -> [w346]
        tunnel: [w345] -> w260
        tunnel: [w344] -> w252
        tunnel: w251 -> [w344]
        tunnel: [w343] -> w249
        tunnel: w248 -> [w343]
        tunnel: [w342] -> w210
        tunnel: w209 -> [w342]
        tunnel: w202 -> [w341]
        tunnel: [w341] -> w201
        tunnel: w260 -> [w359]
        tunnel: [w358] -> w222
        tunnel: [w357] -> w221
        tunnel: w252 -> [w357]
        tunnel: [w354] -> w219
        tunnel: w249 -> [w353]
        tunnel: [w352] -> w211
        tunnel: w210 -> [w352]
        tunnel: w201 -> [w351]
        tunnel: [w351] -> w200
        tunnel: w222 -> [w371]
        tunnel: w221 -> [w376]
        tunnel: [w376] -> w220
        tunnel: w219 -> [w367]
        tunnel: [w366] -> w218
        tunnel: [w370] -> w217
        tunnel: [w365] -> w212
        tunnel: w211 -> [w365]
        tunnel: w200 -> [w364]
        tunnel: [w364] -> w199
        tunnel: [w384] -> w259
        tunnel: [w383] -> w253
        tunnel: w220 -> [w383]
        tunnel: w218 -> [w380]
        tunnel: [w379] -> w233
        tunnel: w217 -> [w385]
        tunnel: [w378] -> w213
        tunnel: w212 -> [w378]
        tunnel: w199 -> [w377]
        tunnel: [w377] -> w198
        tunnel: w259 -> [w398]
        tunnel: [w397] -> w258
        tunnel: [w396] -> w254
        tunnel: w253 -> [w396]
        tunnel: w233 -> [w393]
        tunnel: [w392] -> w224
        tunnel: [w391] -> w214
        tunnel: w213 -> [w391]
        tunnel: w198 -> [w390]
        tunnel: [w390] -> w197
        tunnel: w258 -> [w411]
        tunnel: [w410] -> w257
        tunnel: [w409] -> w255
        tunnel: w254 -> [w409]
        tunnel: w224 -> [w406]
        tunnel: [w405] -> w223
        tunnel: [w404] -> w215
        tunnel: w214 -> [w404]
        tunnel: w197 -> [w403]
        tunnel: [w403] -> w196
        tunnel: w257 -> [w426]
        tunnel: [w425] -> w256
        tunnel: w255 -> [w422]
        tunnel: [w421] -> w228
        tunnel: w223 -> [w418]
        tunnel: [w417] -> w216
        tunnel: w215 -> [w417]
        tunnel: w196 -> [w416]
        tunnel: [w416] -> w195
        tunnel: w256 -> [w438]
        tunnel: [w437] -> w229
        tunnel: w228 -> [w434]
        tunnel: w216 -> [w432]
        tunnel: w195 -> [w431]
        frame #0 {
          n91 = while {
            tunnel: w278 -> [w302]
            tunnel: w277 -> [w297]
            tunnel: [w288] -> w276
            tunnel: w275 -> [w282]
            stop <- TRUE stop-if-true
            # "Drive 20% Speed"
            n92 = call <vilib>:"WPI_EncoderGet.vi"("EncoderDevRef"=w302) -> ("Distance"=w300:dbl)  [unwired: 5 in, 5 out]
            n93 = call <vilib>:"WPI_EncoderGet.vi"("EncoderDevRef"=w282) -> ("Distance"=w287:dbl)  [unwired: 5 in, 5 out]
            n94 = Wait (ms)(milliseconds to wait=u32 10) -> ()  [unwired: 1 out]
            n95 = Absolute Value(x=w300) -> (abs(x)=w299:dbl)
            n96 = Absolute Value(x=w287) -> (abs(x)=w286:dbl)
            n97 = Less?(x=w299, y=20.0) -> (x < y?=w290:bool)
            n98 = Less?(x=w286, y=5.0) -> (x < y?=w283:bool)
            n99 = Select(t=0.2, s=w290, f=0.0) -> (s? t:f=w296:dbl)
            n100 = Select(t=0.2, s=w283, f=0.0) -> ()  [unwired: 1 out]
            n101 = call-poly <vilib>:"WPI_RobotDriveHolonomicDrive.vi"("Rotation"=0.0, "Y"=w296, "X"=0.0, "RobotDriveDevRef"=w297) -> ("error out"=w291:errorcluster, "RobotDriveDevRef"=w288:T12)  [unwired: 5 in, 1 out]
            n102 = flat-sequence {
              tunnel: w291 -> [_]
              tunnel: w290 -> [w304]
              tunnel: [w303] -> _
              frame #0 {
                n103 = Not(x=w304) -> (.not. x?=w303:bool)
              }
            }
          }
          n104 = call-poly <vilib>:"WPI_SolenoidSet.vi"("error in (no error)"=w274, "Value"=WPI_SolenoidValue."Reverse", "SolenoidDevRef"=w273) -> ("error out"=w270:errorcluster, "SolenoidDevRef"=w271:T18)  [unwired: 7 in]
        }
        frame #1 {
          # "Drive Back"
          # "1.25 Second"
          n105 = call-poly <vilib>:"WPI_RobotDriveHolonomicDrive.vi"("Rotation"=0.0, "Y"=0.25, "X"=0.0, "RobotDriveDevRef"=w313) -> ("RobotDriveDevRef"=w310:T12)  [unwired: 5 in, 2 out]
          n106 = Wait (ms)(milliseconds to wait=u32 1250) -> ()  [unwired: 1 out]
        }
        frame #2 {
          w321 = T13 0 items=["PercentOutput"=0, "Position"=1, "Velocity"=2, "Current"=3, "Follower"=5, "MotionProfile"=6, "MotionMagic"=7, "MotionProfileArc"=10, "Disabled"=15] ("Control Mode")
          # "stop and shoot"
          # "1 Second"
          n107 = Wait (ms)(milliseconds to wait=u32 1000) -> ()  [unwired: 1 out]
          n108 = call-poly <vilib>:"WPI_RobotDriveHolonomicDrive.vi"("Rotation"=0.0 ("X axis value"), "Y"=0.0 ("X axis value"), "X"=0.0 ("X axis value"), "RobotDriveDevRef"=w324) -> ("RobotDriveDevRef"=w323:T12)  [unwired: 5 in, 2 out]
          n109 = call <vilib>:"CTRE_Phoenix_MotorControl_Set.vi"("Output"=-1.0, "Control Mode"=w321, "PhoenixMotorControlDevRef"=w319) -> ("PhoenixMotorControlDevRef"=w318:T7)  [unwired: 7 in, 1 out]
        }
        frame #3 {
          w333 = T13 0 items=["PercentOutput"=0, "Position"=1, "Velocity"=2, "Current"=3, "Follower"=5, "MotionProfile"=6, "MotionMagic"=7, "MotionProfileArc"=10, "Disabled"=15] ("Control Mode")
          # "1 Second"
          # "Go foward"
          n110 = call-poly <vilib>:"WPI_RobotDriveHolonomicDrive.vi"("Rotation"=0.0, "Y"=-0.25, "X"=0.0, "RobotDriveDevRef"=w337) -> ("RobotDriveDevRef"=w335:T12)  [unwired: 5 in, 2 out]
          n111 = Wait (ms)(milliseconds to wait=u32 1000) -> ()  [unwired: 1 out]
          n112 = call <vilib>:"CTRE_Phoenix_MotorControl_Set.vi"("Output"=0.0, "Control Mode"=w333, "PhoenixMotorControlDevRef"=w331) -> ("PhoenixMotorControlDevRef"=w330:T7)  [unwired: 7 in, 1 out]
        }
        frame #4 {
          # ".25 Seconds"
          # "Turn"
          n113 = Wait (ms)(milliseconds to wait=u32 250) -> ()  [unwired: 1 out]
          n114 = call-poly <vilib>:"WPI_RobotDriveHolonomicDrive.vi"("Rotation"=0.25, "Y"=0.0, "X"=0.0, "RobotDriveDevRef"=w346) -> ("RobotDriveDevRef"=w345:T12)  [unwired: 5 in, 2 out]
        }
        frame #5 {
          w356 = T13 0 items=["PercentOutput"=0, "Position"=1, "Velocity"=2, "Current"=3, "Follower"=5, "MotionProfile"=6, "MotionMagic"=7, "MotionProfileArc"=10, "Disabled"=15] ("Control Mode")
          # "1 Second"
          # "Go foward"
          n115 = call-poly <vilib>:"WPI_RobotDriveHolonomicDrive.vi"("Rotation"=0.0, "Y"=-0.25, "X"=0.0, "RobotDriveDevRef"=w359) -> ("RobotDriveDevRef"=w358:T12)  [unwired: 5 in, 2 out]
          n116 = Wait (ms)(milliseconds to wait=u32 1000) -> ()  [unwired: 1 out]
          n117 = call <vilib>:"CTRE_Phoenix_MotorControl_Set.vi"("Output"=-1.0, "Control Mode"=w356, "PhoenixMotorControlDevRef"=w353) -> ("PhoenixMotorControlDevRef"=w354:T7)  [unwired: 7 in, 1 out]
        }
        frame #6 {
          w369 = T13 0 items=["PercentOutput"=0, "Position"=1, "Velocity"=2, "Current"=3, "Follower"=5, "MotionProfile"=6, "MotionMagic"=7, "MotionProfileArc"=10, "Disabled"=15] ("Control Mode")
          # "2 Seconds"
          # "Just Intake"
          n118 = call-poly <vilib>:"WPI_RobotDriveHolonomicDrive.vi"("Rotation"=0.0, "Y"=0.0, "X"=0.0, "RobotDriveDevRef"=w371) -> ("RobotDriveDevRef"=w370:T12)  [unwired: 5 in, 2 out]
          n119 = Wait (ms)(milliseconds to wait=u32 2000) -> ()  [unwired: 1 out]
          n120 = call <vilib>:"CTRE_Phoenix_MotorControl_Set.vi"("Output"=-1.0, "Control Mode"=w369, "PhoenixMotorControlDevRef"=w367) -> ("PhoenixMotorControlDevRef"=w366:T7)  [unwired: 7 in, 1 out]
        }
        frame #7 {
          w382 = T13 0 items=["PercentOutput"=0, "Position"=1, "Velocity"=2, "Current"=3, "Follower"=5, "MotionProfile"=6, "MotionMagic"=7, "MotionProfileArc"=10, "Disabled"=15] ("Control Mode")
          # "1 Second"
          # "Go back"
          n121 = call-poly <vilib>:"WPI_RobotDriveHolonomicDrive.vi"("Rotation"=0.0, "Y"=0.25, "X"=0.0, "RobotDriveDevRef"=w385) -> ("RobotDriveDevRef"=w384:T12)  [unwired: 5 in, 2 out]
          n122 = Wait (ms)(milliseconds to wait=u32 1000) -> ()  [unwired: 1 out]
          n123 = call <vilib>:"CTRE_Phoenix_MotorControl_Set.vi"("Output"=-1.0, "Control Mode"=w382, "PhoenixMotorControlDevRef"=w380) -> ("PhoenixMotorControlDevRef"=w379:T7)  [unwired: 7 in, 1 out]
        }
        frame #8 {
          w395 = T13 0 items=["PercentOutput"=0, "Position"=1, "Velocity"=2, "Current"=3, "Follower"=5, "MotionProfile"=6, "MotionMagic"=7, "MotionProfileArc"=10, "Disabled"=15] ("Control Mode")
          # ".25 Seconds"
          # "Turn"
          n124 = call-poly <vilib>:"WPI_RobotDriveHolonomicDrive.vi"("Rotation"=-0.25, "Y"=0.0, "X"=0.0, "RobotDriveDevRef"=w398) -> ("RobotDriveDevRef"=w397:T12)  [unwired: 5 in, 2 out]
          n125 = Wait (ms)(milliseconds to wait=u32 250) -> ()  [unwired: 1 out]
          n126 = call <vilib>:"CTRE_Phoenix_MotorControl_Set.vi"("Output"=-1.0, "Control Mode"=w395, "PhoenixMotorControlDevRef"=w393) -> ("PhoenixMotorControlDevRef"=w392:T7)  [unwired: 7 in, 1 out]
        }
        frame #9 {
          w408 = T13 0 items=["PercentOutput"=0, "Position"=1, "Velocity"=2, "Current"=3, "Follower"=5, "MotionProfile"=6, "MotionMagic"=7, "MotionProfileArc"=10, "Disabled"=15] ("Control Mode")
          # "1 Second"
          # "Go Back"
          n127 = call-poly <vilib>:"WPI_RobotDriveHolonomicDrive.vi"("Rotation"=0.0, "Y"=0.25, "X"=0.0, "RobotDriveDevRef"=w411) -> ("RobotDriveDevRef"=w410:T12)  [unwired: 5 in, 2 out]
          n128 = Wait (ms)(milliseconds to wait=u32 1000) -> ()  [unwired: 1 out]
          n129 = call <vilib>:"CTRE_Phoenix_MotorControl_Set.vi"("Output"=-1.0, "Control Mode"=w408, "PhoenixMotorControlDevRef"=w406) -> ("PhoenixMotorControlDevRef"=w405:T7)  [unwired: 7 in, 1 out]
        }
        frame #10 {
          w420 = T13 0 items=["PercentOutput"=0, "Position"=1, "Velocity"=2, "Current"=3, "Follower"=5, "MotionProfile"=6, "MotionMagic"=7, "MotionProfileArc"=10, "Disabled"=15] ("Control Mode")
          w424 = T13 0 items=["PercentOutput"=0, "Position"=1, "Velocity"=2, "Current"=3, "Follower"=5, "MotionProfile"=6, "MotionMagic"=7, "MotionProfileArc"=10, "Disabled"=15] ("Control Mode")
          # "2 Seconds"
          # "Shoot"
          n130 = call-poly <vilib>:"WPI_RobotDriveHolonomicDrive.vi"("Rotation"=0.0, "Y"=0.0, "X"=0.0, "RobotDriveDevRef"=w426) -> ("RobotDriveDevRef"=w425:T12)  [unwired: 5 in, 2 out]
          n131 = Wait (ms)(milliseconds to wait=u32 2000) -> ()  [unwired: 1 out]
          n132 = call <vilib>:"CTRE_Phoenix_MotorControl_Set.vi"("Output"=-1.0, "Control Mode"=w424, "PhoenixMotorControlDevRef"=w422) -> ("PhoenixMotorControlDevRef"=w421:T7)  [unwired: 7 in, 1 out]
          n133 = call <vilib>:"CTRE_Phoenix_MotorControl_Set.vi"("Output"=0.0, "Control Mode"=w420, "PhoenixMotorControlDevRef"=w418) -> ()  [unwired: 7 in, 2 out]
        }
        frame #11 {
          w436 = T13 0 items=["PercentOutput"=0, "Position"=1, "Velocity"=2, "Current"=3, "Follower"=5, "MotionProfile"=6, "MotionMagic"=7, "MotionProfileArc"=10, "Disabled"=15] ("Control Mode")
          # "2.5 Seconds"
          # "Go foward taxi"
          n134 = call-poly <vilib>:"WPI_RobotDriveHolonomicDrive.vi"("Rotation"=0.0, "Y"=-0.25, "X"=0.0, "RobotDriveDevRef"=w438) -> ("RobotDriveDevRef"=w437:T12)  [unwired: 5 in, 2 out]
          n135 = Wait (ms)(milliseconds to wait=u32 2500) -> ()  [unwired: 1 out]
          n136 = call-poly <vilib>:"WPI_SolenoidSet.vi"("error in (no error)"=w431, "Value"=WPI_SolenoidValue."Forward", "SolenoidDevRef"=w432) -> ()  [unwired: 7 in, 2 out]
          n137 = call <vilib>:"CTRE_Phoenix_MotorControl_Set.vi"("Output"=0.0, "Control Mode"=w436, "PhoenixMotorControlDevRef"=w434) -> ()  [unwired: 7 in, 2 out]
        }
      }
      n138 = call-poly <vilib>:"WPI_RobotDriveHolonomicDrive.vi"("Rotation"=0.0 ("X axis value"), "Y"=0.0 ("X axis value"), "X"=0.0 ("X axis value"), "RobotDriveDevRef"=w229) -> ()  [unwired: 5 in, 3 out]
    }
    frame "Shoot 2 Right side" {
      # "11"
      # "0"
      # "Stand Still"
      # "10"
      # "9"
      # "8"
      # "7"
      # "6"
      # "5"
      # "4"
      # "3"
      # "2"
      # "1"
      # "This sample code describes robot movements in an array. You can extend it to control other motors\non your robot. You can also use file I/O to move the data to a text file."
      n139 = call <vilib>:"WPI_EncoderRefNum Registry Get.vi"("refnum name"="Right Encoder") -> ("EncoderDevRef"=w483:T14)  [unwired: 9 in, 1 out]
      n140 = call <vilib>:"WPI_RobotDriveRefNum Registry Get.vi"("refnum name"="Mecanum Motors") -> ("RobotDriveDevRef"=w486:T12)  [unwired: 1 in, 9 out]
      n141 = call <vilib>:"WPI_EncoderRefNum Registry Get.vi"("refnum name"="Left Encoder") -> ("EncoderDevRef"=w491:T14)  [unwired: 9 in, 1 out]
      n142 = call <vilib>:"CTRE_Phoenix_MotorControl_RefNumRegistryGet.vi"("refnum name"="Indexer") -> ("PhoenixMotorControlDevRef"=w513:T7)  [unwired: 9 in, 1 out]
      n143 = call <vilib>:"CTRE_Phoenix_MotorControl_RefNumRegistryGet.vi"("refnum name"="intake_motor") -> ("PhoenixMotorControlDevRef"=w510:T7)  [unwired: 9 in, 1 out]
      n144 = call <vilib>:"WPI_SolenoidRefNum Registry Get.vi"("refnum name"="intake_cylinder") -> ("error out"=w475:errorcluster, "SolenoidDevRef"=w473:T18)  [unwired: 9 in]
      n145 = call <vilib>:"WPI_EncoderReset.vi"("EncoderDevRef"=w483) -> ("EncoderDevRef"=w482:T14)  [unwired: 9 in, 1 out]
      n146 = call <vilib>:"WPI_RobotDriveSafetyConfig.vi"("mode"=WPI_SafetyOutputConfigMenu."Disable", "RobotDriveDevRef"=w486) -> ("RobotDriveDevRef"=w485:T12)  [unwired: 8 in, 1 out]
      n147 = call <vilib>:"WPI_EncoderReset.vi"("EncoderDevRef"=w491) -> ("EncoderDevRef"=w490:T14)  [unwired: 9 in, 1 out]
      n148 = flat-sequence {
        tunnel: w510 -> [w527]
        tunnel: w513 -> [w528]
        tunnel: [w524] -> w494
        tunnel: [w528] -> w493
        tunnel: [w527] -> w492
        tunnel: w490 -> [w526]
        tunnel: w485 -> [w525]
        tunnel: w482 -> [w523]
        tunnel: w475 -> [w522]
        tunnel: w473 -> [w521]
        tunnel: [w519] -> w464
        tunnel: [w518] -> w443
        tunnel: [w558] -> w517
        tunnel: [w556] -> w514
        tunnel: [w555] -> w511
        tunnel: w494 -> [w561]
        tunnel: w493 -> [w556]
        tunnel: w492 -> [w555]
        tunnel: w464 -> [w554]
        tunnel: [w554] -> w463
        tunnel: [w553] -> w444
        tunnel: w443 -> [w553]
        tunnel: w517 -> [w572]
        tunnel: [w571] -> w516
        tunnel: w514 -> [w567]
        tunnel: w511 -> [w565]
        tunnel: [w566] -> w498
        tunnel: [w565] -> w495
        tunnel: w463 -> [w564]
        tunnel: [w564] -> w462
        tunnel: [w563] -> w445
        tunnel: w444 -> [w563]
        tunnel: w516 -> [w585]
        tunnel: [w583] -> w509
        tunnel: [w578] -> w499
        tunnel: w498 -> [w579]
        tunnel: [w582] -> w496
        tunnel: w495 -> [w582]
        tunnel: w462 -> [w577]
        tunnel: [w577] -> w461
        tunnel: [w576] -> w446
        tunnel: w445 -> [w576]
        tunnel: w509 -> [w594]
        tunnel: [w593] -> w508
        tunnel: [w592] -> w500
        tunnel: w499 -> [w592]
        tunnel: [w591] -> w497
        tunnel: w496 -> [w591]
        tunnel: w461 -> [w590]
        tunnel: [w590] -> w460
        tunnel: [w589] -> w447
        tunnel: w446 -> [w589]
        tunnel: w508 -> [w607]
        tunnel: [w606] -> w470
        tunnel: [w605] -> w469
        tunnel: w500 -> [w605]
        tunnel: [w602] -> w467
        tunnel: w497 -> [w601]
        tunnel: w460 -> [w600]
        tunnel: [w600] -> w459
        tunnel: [w599] -> w448
        tunnel: w447 -> [w599]
        tunnel: w470 -> [w619]
        tunnel: w469 -> [w624]
        tunnel: [w624] -> w468
        tunnel: w467 -> [w615]
        tunnel: [w614] -> w466
        tunnel: [w618] -> w465
        tunnel: w459 -> [w613]
        tunnel: [w613] -> w458
        tunnel: [w612] -> w449
        tunnel: w448 -> [w612]
        tunnel: [w632] -> w507
        tunnel: [w631] -> w501
        tunnel: w468 -> [w631]
        tunnel: w466 -> [w628]
        tunnel: [w627] -> w481
        tunnel: w465 -> [w633]
        tunnel: w458 -> [w626]
        tunnel: [w626] -> w457
        tunnel: [w625] -> w450
        tunnel: w449 -> [w625]
        tunnel: w507 -> [w646]
        tunnel: [w645] -> w506
        tunnel: [w644] -> w502
        tunnel: w501 -> [w644]
        tunnel: w481 -> [w641]
        tunnel: [w640] -> w472
        tunnel: w457 -> [w639]
        tunnel: [w639] -> w456
        tunnel: [w638] -> w451
        tunnel: w450 -> [w638]
        tunnel: w506 -> [w659]
        tunnel: [w658] -> w505
        tunnel: [w657] -> w503
        tunnel: w502 -> [w657]
        tunnel: w472 -> [w654]
        tunnel: [w653] -> w471
        tunnel: w456 -> [w652]
        tunnel: [w652] -> w455
        tunnel: [w651] -> w452
        tunnel: w451 -> [w651]
        tunnel: w505 -> [w674]
        tunnel: [w673] -> w504
        tunnel: w503 -> [w670]
        tunnel: [w669] -> w476
        tunnel: w471 -> [w666]
        tunnel: w455 -> [w665]
        tunnel: [w665] -> w454
        tunnel: [w664] -> w453
        tunnel: w452 -> [w664]
        tunnel: w504 -> [w686]
        tunnel: [w685] -> w477
        tunnel: w476 -> [w682]
        tunnel: w454 -> [w680]
        tunnel: w453 -> [w679]
        frame #0 {
          n149 = while {
            tunnel: w526 -> [w550]
            tunnel: w525 -> [w545]
            tunnel: [w536] -> w524
            tunnel: w523 -> [w530]
            stop <- TRUE stop-if-true
            # "Drive 20% Speed"
            n150 = call <vilib>:"WPI_EncoderGet.vi"("EncoderDevRef"=w550) -> ("Distance"=w548:dbl)  [unwired: 5 in, 5 out]
            n151 = call <vilib>:"WPI_EncoderGet.vi"("EncoderDevRef"=w530) -> ("Distance"=w535:dbl)  [unwired: 5 in, 5 out]
            n152 = Wait (ms)(milliseconds to wait=u32 10) -> ()  [unwired: 1 out]
            n153 = Absolute Value(x=w548) -> (abs(x)=w547:dbl)
            n154 = Absolute Value(x=w535) -> (abs(x)=w534:dbl)
            n155 = Less?(x=w547, y=20.0) -> (x < y?=w538:bool)
            n156 = Less?(x=w534, y=5.0) -> (x < y?=w531:bool)
            n157 = Select(t=0.2, s=w538, f=0.0) -> (s? t:f=w544:dbl)
            n158 = Select(t=0.2, s=w531, f=0.0) -> ()  [unwired: 1 out]
            n159 = call-poly <vilib>:"WPI_RobotDriveHolonomicDrive.vi"("Rotation"=0.0, "Y"=w544, "X"=0.0, "RobotDriveDevRef"=w545) -> ("error out"=w539:errorcluster, "RobotDriveDevRef"=w536:T12)  [unwired: 5 in, 1 out]
            n160 = flat-sequence {
              tunnel: w539 -> [_]
              tunnel: w538 -> [w552]
              tunnel: [w551] -> _
              frame #0 {
                n161 = Not(x=w552) -> (.not. x?=w551:bool)
              }
            }
          }
          n162 = call-poly <vilib>:"WPI_SolenoidSet.vi"("error in (no error)"=w522, "Value"=WPI_SolenoidValue."Reverse", "SolenoidDevRef"=w521) -> ("error out"=w518:errorcluster, "SolenoidDevRef"=w519:T18)  [unwired: 7 in]
        }
        frame #1 {
          # "Drive Back"
          # "1.25 Second"
          n163 = call-poly <vilib>:"WPI_RobotDriveHolonomicDrive.vi"("Rotation"=0.0, "Y"=0.25, "X"=0.0, "RobotDriveDevRef"=w561) -> ("RobotDriveDevRef"=w558:T12)  [unwired: 5 in, 2 out]
          n164 = Wait (ms)(milliseconds to wait=u32 1250) -> ()  [unwired: 1 out]
        }
        frame #2 {
          w569 = T13 0 items=["PercentOutput"=0, "Position"=1, "Velocity"=2, "Current"=3, "Follower"=5, "MotionProfile"=6, "MotionMagic"=7, "MotionProfileArc"=10, "Disabled"=15] ("Control Mode")
          # "stop and shoot"
          # "1 Second"
          n165 = Wait (ms)(milliseconds to wait=u32 1000) -> ()  [unwired: 1 out]
          n166 = call-poly <vilib>:"WPI_RobotDriveHolonomicDrive.vi"("Rotation"=0.0 ("X axis value"), "Y"=0.0 ("X axis value"), "X"=0.0 ("X axis value"), "RobotDriveDevRef"=w572) -> ("RobotDriveDevRef"=w571:T12)  [unwired: 5 in, 2 out]
          n167 = call <vilib>:"CTRE_Phoenix_MotorControl_Set.vi"("Output"=-1.0, "Control Mode"=w569, "PhoenixMotorControlDevRef"=w567) -> ("PhoenixMotorControlDevRef"=w566:T7)  [unwired: 7 in, 1 out]
        }
        frame #3 {
          w581 = T13 0 items=["PercentOutput"=0, "Position"=1, "Velocity"=2, "Current"=3, "Follower"=5, "MotionProfile"=6, "MotionMagic"=7, "MotionProfileArc"=10, "Disabled"=15] ("Control Mode")
          # "1 Second"
          # "Go foward"
          n168 = call-poly <vilib>:"WPI_RobotDriveHolonomicDrive.vi"("Rotation"=0.0, "Y"=-0.25, "X"=0.0, "RobotDriveDevRef"=w585) -> ("RobotDriveDevRef"=w583:T12)  [unwired: 5 in, 2 out]
          n169 = Wait (ms)(milliseconds to wait=u32 1000) -> ()  [unwired: 1 out]
          n170 = call <vilib>:"CTRE_Phoenix_MotorControl_Set.vi"("Output"=0.0, "Control Mode"=w581, "PhoenixMotorControlDevRef"=w579) -> ("PhoenixMotorControlDevRef"=w578:T7)  [unwired: 7 in, 1 out]
        }
        frame #4 {
          # ".25 Seconds"
          # "Turn"
          n171 = Wait (ms)(milliseconds to wait=u32 250) -> ()  [unwired: 1 out]
          n172 = call-poly <vilib>:"WPI_RobotDriveHolonomicDrive.vi"("Rotation"=-0.25, "Y"=0.0, "X"=0.0, "RobotDriveDevRef"=w594) -> ("RobotDriveDevRef"=w593:T12)  [unwired: 5 in, 2 out]
        }
        frame #5 {
          w604 = T13 0 items=["PercentOutput"=0, "Position"=1, "Velocity"=2, "Current"=3, "Follower"=5, "MotionProfile"=6, "MotionMagic"=7, "MotionProfileArc"=10, "Disabled"=15] ("Control Mode")
          # "1 Second"
          # "Go foward"
          n173 = call-poly <vilib>:"WPI_RobotDriveHolonomicDrive.vi"("Rotation"=0.0, "Y"=-0.25, "X"=0.0, "RobotDriveDevRef"=w607) -> ("RobotDriveDevRef"=w606:T12)  [unwired: 5 in, 2 out]
          n174 = Wait (ms)(milliseconds to wait=u32 1000) -> ()  [unwired: 1 out]
          n175 = call <vilib>:"CTRE_Phoenix_MotorControl_Set.vi"("Output"=-1.0, "Control Mode"=w604, "PhoenixMotorControlDevRef"=w601) -> ("PhoenixMotorControlDevRef"=w602:T7)  [unwired: 7 in, 1 out]
        }
        frame #6 {
          w617 = T13 0 items=["PercentOutput"=0, "Position"=1, "Velocity"=2, "Current"=3, "Follower"=5, "MotionProfile"=6, "MotionMagic"=7, "MotionProfileArc"=10, "Disabled"=15] ("Control Mode")
          # "2 Seconds"
          # "Just Intake"
          n176 = call-poly <vilib>:"WPI_RobotDriveHolonomicDrive.vi"("Rotation"=0.0, "Y"=0.0, "X"=0.0, "RobotDriveDevRef"=w619) -> ("RobotDriveDevRef"=w618:T12)  [unwired: 5 in, 2 out]
          n177 = Wait (ms)(milliseconds to wait=u32 2000) -> ()  [unwired: 1 out]
          n178 = call <vilib>:"CTRE_Phoenix_MotorControl_Set.vi"("Output"=-1.0, "Control Mode"=w617, "PhoenixMotorControlDevRef"=w615) -> ("PhoenixMotorControlDevRef"=w614:T7)  [unwired: 7 in, 1 out]
        }
        frame #7 {
          w630 = T13 0 items=["PercentOutput"=0, "Position"=1, "Velocity"=2, "Current"=3, "Follower"=5, "MotionProfile"=6, "MotionMagic"=7, "MotionProfileArc"=10, "Disabled"=15] ("Control Mode")
          # "1 Second"
          # "Go back"
          n179 = call-poly <vilib>:"WPI_RobotDriveHolonomicDrive.vi"("Rotation"=0.0, "Y"=0.25, "X"=0.0, "RobotDriveDevRef"=w633) -> ("RobotDriveDevRef"=w632:T12)  [unwired: 5 in, 2 out]
          n180 = Wait (ms)(milliseconds to wait=u32 1000) -> ()  [unwired: 1 out]
          n181 = call <vilib>:"CTRE_Phoenix_MotorControl_Set.vi"("Output"=-1.0, "Control Mode"=w630, "PhoenixMotorControlDevRef"=w628) -> ("PhoenixMotorControlDevRef"=w627:T7)  [unwired: 7 in, 1 out]
        }
        frame #8 {
          w643 = T13 0 items=["PercentOutput"=0, "Position"=1, "Velocity"=2, "Current"=3, "Follower"=5, "MotionProfile"=6, "MotionMagic"=7, "MotionProfileArc"=10, "Disabled"=15] ("Control Mode")
          # ".25 Seconds"
          # "Turn"
          n182 = call-poly <vilib>:"WPI_RobotDriveHolonomicDrive.vi"("Rotation"=0.25, "Y"=0.0, "X"=0.0, "RobotDriveDevRef"=w646) -> ("RobotDriveDevRef"=w645:T12)  [unwired: 5 in, 2 out]
          n183 = Wait (ms)(milliseconds to wait=u32 250) -> ()  [unwired: 1 out]
          n184 = call <vilib>:"CTRE_Phoenix_MotorControl_Set.vi"("Output"=-1.0, "Control Mode"=w643, "PhoenixMotorControlDevRef"=w641) -> ("PhoenixMotorControlDevRef"=w640:T7)  [unwired: 7 in, 1 out]
        }
        frame #9 {
          w656 = T13 0 items=["PercentOutput"=0, "Position"=1, "Velocity"=2, "Current"=3, "Follower"=5, "MotionProfile"=6, "MotionMagic"=7, "MotionProfileArc"=10, "Disabled"=15] ("Control Mode")
          # "1 Second"
          # "Go Back"
          n185 = call-poly <vilib>:"WPI_RobotDriveHolonomicDrive.vi"("Rotation"=0.0, "Y"=0.25, "X"=0.0, "RobotDriveDevRef"=w659) -> ("RobotDriveDevRef"=w658:T12)  [unwired: 5 in, 2 out]
          n186 = Wait (ms)(milliseconds to wait=u32 1000) -> ()  [unwired: 1 out]
          n187 = call <vilib>:"CTRE_Phoenix_MotorControl_Set.vi"("Output"=-1.0, "Control Mode"=w656, "PhoenixMotorControlDevRef"=w654) -> ("PhoenixMotorControlDevRef"=w653:T7)  [unwired: 7 in, 1 out]
        }
        frame #10 {
          w668 = T13 0 items=["PercentOutput"=0, "Position"=1, "Velocity"=2, "Current"=3, "Follower"=5, "MotionProfile"=6, "MotionMagic"=7, "MotionProfileArc"=10, "Disabled"=15] ("Control Mode")
          w672 = T13 0 items=["PercentOutput"=0, "Position"=1, "Velocity"=2, "Current"=3, "Follower"=5, "MotionProfile"=6, "MotionMagic"=7, "MotionProfileArc"=10, "Disabled"=15] ("Control Mode")
          # "2 Seconds"
          # "Shoot"
          n188 = call-poly <vilib>:"WPI_RobotDriveHolonomicDrive.vi"("Rotation"=0.0, "Y"=0.0, "X"=0.0, "RobotDriveDevRef"=w674) -> ("RobotDriveDevRef"=w673:T12)  [unwired: 5 in, 2 out]
          n189 = Wait (ms)(milliseconds to wait=u32 2000) -> ()  [unwired: 1 out]
          n190 = call <vilib>:"CTRE_Phoenix_MotorControl_Set.vi"("Output"=-1.0, "Control Mode"=w672, "PhoenixMotorControlDevRef"=w670) -> ("PhoenixMotorControlDevRef"=w669:T7)  [unwired: 7 in, 1 out]
          n191 = call <vilib>:"CTRE_Phoenix_MotorControl_Set.vi"("Output"=0.0, "Control Mode"=w668, "PhoenixMotorControlDevRef"=w666) -> ()  [unwired: 7 in, 2 out]
        }
        frame #11 {
          w684 = T13 0 items=["PercentOutput"=0, "Position"=1, "Velocity"=2, "Current"=3, "Follower"=5, "MotionProfile"=6, "MotionMagic"=7, "MotionProfileArc"=10, "Disabled"=15] ("Control Mode")
          # "2.5 Seconds"
          # "Go foward taxi"
          n192 = call-poly <vilib>:"WPI_RobotDriveHolonomicDrive.vi"("Rotation"=0.0, "Y"=-0.25, "X"=0.0, "RobotDriveDevRef"=w686) -> ("RobotDriveDevRef"=w685:T12)  [unwired: 5 in, 2 out]
          n193 = Wait (ms)(milliseconds to wait=u32 2500) -> ()  [unwired: 1 out]
          n194 = call-poly <vilib>:"WPI_SolenoidSet.vi"("error in (no error)"=w679, "Value"=WPI_SolenoidValue."Forward", "SolenoidDevRef"=w680) -> ()  [unwired: 7 in, 2 out]
          n195 = call <vilib>:"CTRE_Phoenix_MotorControl_Set.vi"("Output"=0.0, "Control Mode"=w684, "PhoenixMotorControlDevRef"=w682) -> ()  [unwired: 7 in, 2 out]
        }
      }
      n196 = call-poly <vilib>:"WPI_RobotDriveHolonomicDrive.vi"("Rotation"=0.0 ("X axis value"), "Y"=0.0 ("X axis value"), "X"=0.0 ("X axis value"), "RobotDriveDevRef"=w477) -> ()  [unwired: 5 in, 3 out]
    }
    frame "Your Turn" {
    }
  }
